vi "RT_foursetup.vi"() -> ()   [LabVIEW 2015]
uses:
  <vilib>/Platform/TimedLoop/XDataNode/timing_clust.ctl
  <vilib>/Platform/TimedLoop/XDataNode/nitl_modes.ctl
  <vilib>/Platform/TimedLoop/XDataNode/wakeup.ctl
  <vilib>/FPGAPlugInAG/myRIO-1950/niLvFpga_Open_myRIO-1950.vi
  <vilib>/rvi/interface/common/dynamic/niFpgaDynamicAddResources.vi
  <vilib>/Utility/error.llb/Error Cluster From Error Code.vi
  <vilib>/rvi/errors/niLvFpgaAdjustHostInterfaceError.vi
  <vilib>/RVI Host/nirviSupport.llb/nirviErrorClusterFromErrorCode.vi
  <vilib>/Analysis/3filter.llb/Butterworth Filter (DBL).vi
  <vilib>/rvi/interface/nirviOpenFPGA/nirviOpenFPGA.xnode
  FPGA Bitfiles/Flylaserbox_FPGATarget_FPGALASER4SETUPF_niW-GusbrOo.lvbitx
  FPGA_LASER_4SETUP_Feb19_2016.vi
  <vilib>/rvi/interface/nirviReadWriteControl/nirviReadWriteControl.xnode
  <vilib>/Platform/TimedLoop/XDataNode/XDataNode.xnode
  <vilib>/rvi/interface/nirviMethod/nirviMethod.xnode
  <vilib>/rvi/interface/Simulation/niFpgaSimulationCallBeginRW.vi
  <vilib>/Platform/TimedLoop/XDataNode/XDNodeRunTimeDep.lvlib
  <vilib>/rvi/interface/nirviMethod/StockFPGA_InlinedMethodWaitForSingleIRQ.vi
  <vilib>/FPGAPlugInAG/Dynamic/niLvFpga_WaitOnIrq_Dynamic.vi
  <vilib>/FPGAPlugInAG/Dynamic/niLvFpga_ReadFifo_Dynamic.vi
  <vilib>/rvi/errors/niLvFpgaMergeErrorWithErrorCode.vi
  <vilib>/FPGAPlugInAG/Dynamic/niLvFpga_AcknowledgeIrq_Dynamic.vi
  <vilib>/Analysis/NI_AALBase.lvlib
  NiFpgaLv.dll
panel:
  out "x-y*floor(x/y) 2":u16
  out "x-y*floor(x/y)":u16
  in  "Low Period (ticks) J8":u32
  in  "Low Period (ticks) J4":u32
  in  "Low Period (ticks) J5":u32
  in  "Low Period (ticks) J1":u32
  out "Elements Remaining 8":u32
  out "Elements Remaining 7":u32
  out "Elements Remaining 6":u32
  out "Elements Remaining 5":u32
  out "Elements Remaining 4":u32
  out "Elements Remaining 3":u32
  out "Elements Remaining 2":u32
  out "Elements Remaining":u32
  out "IRQ(s) Asserted 4":i32
  out "IRQ(s) Asserted 3":i32
  out "IRQ(s) Asserted 2":i32
  out "IRQ(s) Asserted":i32
  out "Frame Count":i16=10040
  in  "Manual control for laser":bool
  in  "Laser current control 3":u16=629
  in  "Laser current control 4":u16=629
  in  "Laser current control":u16=583
  in  "Laser current control 2":u16=629
  in  "FPGA Stop":bool
  out "Path 3":path
  out "appended path":path
  out "Path 2":path
  in  "Path":path
  out "Fly real-time location/center mass":dbl(graph)=575.5038458695241
  in  "order":i32=3
  in  "low cutoff freq: fl":dbl=40.0 format="%0.4f"
  in  "high cutoff freq: fh":dbl=400.0 format="%0.2f"
  in  "sampling freq: fs":dbl=1000.0 format="%0.2f"
  in  "threshold 3":dbl=5.0
  in  "control":u16=1
  out "Subtraction-10 frames average":dbl[](graph)=[1120.6666666666665, 1157.0, 1210.6666666666665, 1210.3333333333335, 1269.2222222222222, 1265.2222222222222, 1320.3333333333335, 1302.7777777777778, 1340.5555555555557, 1328.7777777777778, 1360.5555555555557, 1346.0, 1377.5555555555557, 1365.3333333333335, 1395.2222222222222, 1384.0, 1415.0, 1405.0, 1439.0, 1427.3333333333335, 1464.0, 1467.6666666666665, 1525.6666666666665, 1554.7777777777778, 1636.3333333333335, 1657.7777777777778, 1730.4444444444443, 1741.6666666666665, 1801.2222222222222, 1808.888888888889, 1870.3333333333335, 1880.5555555555557, 1940.3333333333335, 1944.0, 2005.0, 2002.2222222222222, 2050.0, 2039.4444444444443, 2086.4444444444443, 2082.4444444444443, 2131.777777777778, 2119.222222222222, 2166.8888888888887, 2155.4444444444443, 2197.0, 2181.8888888888887, 2225.4444444444443, 2205.8888888888887, 2243.1111111111113, 2216.4444444444443, 2259.333333333333, 2237.5555555555557, 2271.4444444444443, 2241.666666666667, 2276.777777777778, 2247.4444444444443, 2285.4444444444443, 2248.777777777778, 2285.222222222222, 2253.4444444444443, 2291.5555555555557, 2259.666666666667, 2290.666666666667, 2268.8888888888887, 2301.777777777778, 2265.4444444444443, 2306.5555555555557, 2273.8888888888887, 2306.777777777778, 2274.1111111111113, 2312.222222222222, 2278.777777777778, 2313.5555555555557, 2280.222222222222, 2316.1111111111113, 2277.666666666667, 2310.8888888888887, 2278.333333333333, 2313.777777777778, 2282.333333333333, 2305.1111111111113, 2272.0, 2304.1111111111113, 2273.333333333333, 2297.5555555555557, 2263.4444444444443, 2289.777777777778, 2257.8888888888887, 2287.0, 2246.333333333333, 2274.333333333333, 2240.4444444444443, 2264.4444444444443, 2228.333333333333, 2253.8888888888887, 2223.8888888888887, 2251.1111111111113, 2217.222222222222, 2247.0, 2214.0, 2238.4444444444443, 2201.222222222222, 2233.8888888888887, 2195.4444444444443, 2223.777777777778, 2188.777777777778, 2216.5555555555557, 2180.5555555555557, 2212.333333333333, 2176.222222222222, 2199.333333333333, 2166.666666666667, 2204.5555555555557, 2169.5555555555557, 2197.4444444444443, 2169.1111111111113, 2202.1111111111113, 2168.5555555555557, 2199.777777777778, 2173.0, 2204.5555555555557, 2160.666666666667, 2201.8888888888887, 2170.777777777778, 2197.1111111111113, 2164.0, 2186.222222222222, 2119.222222222222, 2163.5555555555557, 2179.8888888888887, 2189.4444444444443, 2190.0, 2185.1111111111113, 2187.222222222222, 2181.4444444444443, 2172.4444444444443, 2167.777777777778, 2167.0, 2149.222222222222, 2149.1111111111113, 2149.666666666667, 2153.8888888888887, 2145.0, 2149.8888888888887, 2142.777777777778, 2141.222222222222, 2137.222222222222, 2136.666666666667, 2131.0, 2131.666666666667, 2137.1111111111113, 2142.1111111111113, 2135.777777777778, 2132.666666666667, 2128.1111111111113, 2127.4444444444443, 2121.222222222222, 2122.8888888888887, 2113.4444444444443, 2114.1111111111113, 2088.333333333333, 2099.222222222222, 2110.222222222222, 2112.666666666667, 2110.0, 2112.777777777778, 2102.8888888888887, 2112.4444444444443, 2105.333333333333, 2098.5555555555557, 2103.333333333333, 2105.5555555555557, 2099.333333333333, 2087.666666666667, 2084.333333333333, 2095.4444444444443, 2091.222222222222, 2096.5555555555557, 2099.4444444444443, 2093.777777777778, 2093.333333333333, 2100.1111111111113, 2091.222222222222, 2096.0, 2094.666666666667, 2092.0, 2090.333333333333, 2084.4444444444443, 2082.222222222222, 2086.4444444444443, 2078.222222222222, 2082.0, 2083.8888888888887, 2088.777777777778, 2092.777777777778, 2090.1111111111113, 2088.222222222222, 2086.0, 2086.0, 2094.0, 2090.222222222222, 2093.333333333333, 2089.0, 2090.5555555555557, 2093.5555555555557, 2089.333333333333, 2088.222222222222, 2088.777777777778, 2092.222222222222, 2092.333333333333, 2096.4444444444443, 2096.5555555555557, 2091.5555555555557, 2094.4444444444443, 2094.0, 2095.666666666667, 2092.0, 2100.5555555555557, 2105.1111111111113, 2100.1111111111113, 2097.222222222222, 2098.8888888888887, 2096.5555555555557, 2100.1111111111113, 2107.0, 2102.222222222222, 2102.222222222222, 2097.777777777778, 2098.4444444444443, 2100.777777777778, 2099.777777777778, 2103.222222222222, 2106.4444444444443, 2109.0, 2103.1111111111113, 2110.222222222222, 2113.0, 2107.1111111111113, 2113.777777777778, 2120.0, 2121.333333333333, 2113.666666666667, 2111.0, 2108.1111111111113, 2105.8888888888887, 2105.5555555555557, 2102.8888888888887, 2104.8888888888887, 2104.666666666667, 2100.777777777778, 2105.1111111111113, 2108.5555555555557, 2104.777777777778, 2106.1111111111113, 2096.1111111111113, 2078.222222222222, 1942.888888888889, 1945.888888888889, 1952.5555555555557, 1946.111111111111, 1948.111111111111, 1945.5555555555557, 1953.0, 1959.888888888889, 1950.111111111111, 1938.0, 1953.5555555555557, 1957.2222222222222, 1962.4444444444443, 1957.111111111111, 1960.0, 1953.6666666666665, 1962.0, 1951.111111111111, 1958.0, 1961.2222222222222, 1966.5555555555557, 1967.5555555555557, 1962.3333333333335, 1965.888888888889, 1958.111111111111, 1957.3333333333335, 1957.7777777777778, 1953.2222222222222, 1958.5555555555557, 1961.111111111111, 1958.111111111111, 1963.3333333333335, 1968.0, 1965.2222222222222, 1965.888888888889, 1958.3333333333335, 1962.3333333333335, 1958.2222222222222, 1954.6666666666665, 1943.4444444444443, 1943.7777777777778, 1940.5555555555557, 1938.111111111111, 1924.7777777777778, 1930.3333333333335, 1923.4444444444443, 1914.5555555555557, 1910.111111111111, 1903.2222222222222, 1906.111111111111, 1909.5555555555557, 1894.4444444444443, 1877.6666666666665, 1863.5555555555557, 1862.0, 1839.7777777777778, 1827.2222222222222, 1850.2222222222222, 1859.111111111111, 1852.888888888889, 1870.2222222222222, 1883.888888888889, 1898.7777777777778, 1897.3333333333335, 1894.4444444444443, 1893.2222222222222, 1890.0, 1885.7777777777778, 1889.888888888889, 1893.111111111111, 1901.111111111111, 1896.7777777777778, 1900.888888888889, 1906.888888888889, 1913.888888888889, 1910.5555555555557, 1908.5555555555557, 1905.888888888889, 1906.111111111111, 1905.111111111111, 1908.2222222222222, 1897.6666666666665, 1901.2222222222222, 1904.6666666666665, 1904.0, 1902.111111111111, 1906.4444444444443, 1909.0, 1901.6666666666665, 1894.3333333333335, 1891.7777777777778, 1893.111111111111, 1895.888888888889, 1903.6666666666665, 1905.2222222222222, 1902.6666666666665, 1908.5555555555557, 1900.888888888889, 1902.5555555555557, 1897.7777777777778, 1899.6666666666665, 1896.5555555555557, 1893.4444444444443, 1886.4444444444443, 1888.3333333333335, 1889.3333333333335, 1890.7777777777778, 1891.0, 1892.4444444444443, 1890.0, 1885.0, 1880.6666666666665, 1892.111111111111, 1891.7777777777778, 1892.0, 1895.7777777777778, 1892.2222222222222, 1893.5555555555557, 1899.7777777777778, 1890.111111111111, 1890.2222222222222, 1884.2222222222222, 1884.5555555555557, 1876.2222222222222, 1877.4444444444443, 1864.6666666666665, 1860.2222222222222, 1854.7777777777778, 1946.0, 1928.6666666666665, 1965.2222222222222, 1933.888888888889, 1965.888888888889, 1939.111111111111, 1971.2222222222222, 1940.4444444444443, 1967.4444444444443, 1935.3333333333335, 1968.0, 1935.3333333333335, 1966.0, 1933.2222222222222, 1959.5555555555557, 1925.7777777777778, 1951.0, 1918.4444444444443, 1951.7777777777778, 1927.3333333333335, 1958.888888888889, 1927.3333333333335, 1944.888888888889, 1923.111111111111, 1960.6666666666665, 1925.111111111111, 1964.111111111111, 1931.7777777777778, 1958.888888888889, 1930.0, 1963.2222222222222, 1932.6666666666665, 1956.888888888889, 1924.2222222222222, 1963.6666666666665, 1934.3333333333335, 1958.4444444444443, 1932.6666666666665, 1964.0, 1932.888888888889, 1958.6666666666665, 1932.888888888889, 1964.111111111111, 1934.3333333333335, 1958.111111111111, 1930.4444444444443, 1957.2222222222222, 1928.7777777777778, 1959.3333333333335, 1921.111111111111, 1958.5555555555557, 1924.2222222222222, 1950.0, 1922.111111111111, 1948.888888888889, 1921.3333333333335, 1953.3333333333335, 1922.0, 1953.7777777777778, 1918.4444444444443, 1953.4444444444443, 1920.5555555555557, 1953.5555555555557, 1919.5555555555557, 1947.5555555555557, 1921.5555555555557, 1947.3333333333335, 1921.111111111111, 1941.4444444444443, 1913.111111111111, 1941.888888888889, 1913.7777777777778, 1938.4444444444443, 1896.888888888889, 1926.4444444444443, 1896.5555555555557, 1926.5555555555557, 1897.0, 1923.5555555555557, 1898.7777777777778, 1931.888888888889, 1899.888888888889, 1931.111111111111, 1898.4444444444443, 1934.0, 1899.4444444444443, 1933.3333333333335, 1901.7777777777778, 1937.888888888889, 1901.4444444444443, 1935.2222222222222, 1902.6666666666665, 1934.3333333333335, 1903.2222222222222, 1932.5555555555557, 1912.5555555555557, 1940.888888888889, 1904.5555555555557, 1936.0, 1904.7777777777778, 1939.888888888889, 1921.111111111111, 1938.0, 1912.3333333333335, 1936.7777777777778, 1903.888888888889, 1936.0, 1912.888888888889, 1936.7777777777778, 1904.888888888889, 1945.5555555555557, 1908.4444444444443, 1934.2222222222222, 1908.0, 1935.888888888889, 1906.0, 1934.2222222222222, 1902.4444444444443, 1931.2222222222222, 1908.0, 1938.2222222222222, 1909.0, 1936.3333333333335, 1913.3333333333335, 1945.888888888889, 1911.3333333333335, 1924.6666666666665, 1886.2222222222222, 1883.7777777777778, 1862.111111111111, 1887.6666666666665, 1874.7777777777778, 1902.6666666666665, 1875.111111111111, 1890.2222222222222, 1882.7777777777778, 1908.2222222222222, 1886.5555555555557, 1904.2222222222222, 1889.5555555555557, 1913.5555555555557, 1890.5555555555557, 1913.5555555555557, 1890.5555555555557, 1905.2222222222222, 1883.888888888889, 1912.111111111111, 1888.111111111111, 1913.888888888889, 1886.6666666666665, 1924.888888888889, 1894.0, 1915.5555555555557, 1889.4444444444443, 1910.7777777777778, 1888.5555555555557, 1909.6666666666665, 1894.888888888889, 1921.0, 1905.4444444444443, 1928.0, 1903.3333333333335, 1923.888888888889, 1900.6666666666665, 1922.888888888889, 1905.3333333333335, 1927.4444444444443, 1914.888888888889, 1929.4444444444443, 1908.888888888889, 1928.888888888889, 1901.3333333333335, 1925.0, 1906.7777777777778, 1929.6666666666665, 1908.4444444444443, 1935.888888888889, 1913.111111111111, 1934.3333333333335, 1910.3333333333335, 1927.111111111111, 1906.2222222222222, 1931.5555555555557, 1917.5555555555557, 1944.5555555555557, 1918.5555555555557, 1943.7777777777778, 1924.2222222222222, 1948.3333333333335, 1928.5555555555557, 1953.888888888889, 1937.111111111111, 1964.888888888889, 1943.888888888889, 1966.6666666666665, 1942.6666666666665, 1966.0, 1948.888888888889, 1967.6666666666665, 1942.4444444444443, 1965.3333333333335, 1943.0, 1964.3333333333335, 1949.3333333333335, 1972.7777777777778, 1947.5555555555557, 1973.0, 1950.888888888889, 1979.3333333333335, 1952.6666666666665, 1975.6666666666665, 1961.3333333333335, 1978.4444444444443, 1956.4444444444443, 1978.2222222222222, 1960.3333333333335, 1983.111111111111, 1960.0, 1985.0, 1962.7777777777778, 1984.2222222222222, 1961.7777777777778, 1986.888888888889, 1960.6666666666665, 1984.111111111111, 1958.2222222222222, 1977.6666666666665, 1961.111111111111, 1981.4444444444443, 1960.888888888889, 1980.6666666666665, 1959.6666666666665, 1980.888888888889, 1958.2222222222222, 1977.888888888889, 1961.6666666666665, 1982.3333333333335, 1964.3333333333335, 1990.0, 1972.7777777777778, 1997.3333333333335, 1970.7777777777778, 1996.888888888889, 1972.5555555555557, 1997.3333333333335, 1978.2222222222222, 1998.3333333333335, 1977.2222222222222, 2000.5555555555557, 1977.4444444444443, 2008.5555555555557, 1980.888888888889, 2003.7777777777778, 1991.3333333333335, 2001.4444444444443, 1964.3333333333335, 2019.888888888889, 1998.6666666666665, 2019.2222222222222, 2005.6666666666665, 2021.888888888889, 2013.4444444444443, 2031.111111111111, 2018.4444444444443, 2050.0, 2018.111111111111, 2044.6666666666665, 2021.6666666666665, 2044.4444444444443, 2023.6666666666665, 2050.5555555555557, 2036.2222222222222, 2054.1111111111113, 2031.3333333333335, 2059.5555555555557, 2039.0, 2056.333333333333, 2037.111111111111, 2060.4444444444443, 2049.4444444444443, 2069.8888888888887, 2044.7777777777778, 2071.4444444444443, 2053.333333333333, 2072.222222222222, 2058.4444444444443, 2080.4444444444443, 2064.777777777778, 2090.333333333333, 2067.8888888888887, 2089.333333333333, 2069.666666666667, 2093.0, 2077.666666666667, 2094.777777777778, 2076.4444444444443, 2095.0, 2075.4444444444443, 2096.8888888888887, 2079.777777777778, 2099.777777777778, 2082.5555555555557, 2102.666666666667, 2085.0, 2104.0, 2080.0, 2102.5555555555557, 2080.4444444444443, 2093.8888888888887, 2072.0, 2095.0, 2072.1111111111113, 2083.8888888888887, 2053.5555555555557, 2073.5555555555557, 2042.4444444444443, 2053.666666666667, 2022.6666666666665, 2033.0, 2003.888888888889, 2027.0, 1992.2222222222222, 2003.7777777777778, 1973.0, 1984.7777777777778, 1956.3333333333335, 1968.0, 1937.7777777777778, 1951.7777777777778, 1920.7777777777778, 1929.7777777777778, 1914.111111111111, 1917.2222222222222, 1888.2222222222222, 1889.4444444444443, 1877.7777777777778, 1889.888888888889, 1864.5555555555557, 1879.4444444444443, 1858.6666666666665, 1858.5555555555557, 1820.2222222222222, 1821.4444444444443, 1783.3333333333335, 1779.888888888889, 1742.2222222222222, 1741.2222222222222, 1708.888888888889, 1709.5555555555557, 1681.4444444444443, 1682.0, 1653.5555555555557, 1660.111111111111, 1625.4444444444443, 1620.0, 1574.2222222222222, 1554.2222222222222, 1502.6666666666665, 1484.6666666666665, 1457.3333333333335, 1458.111111111111, 1436.6666666666665, 1441.6666666666665, 1421.7777777777778, 1425.0, 1404.888888888889, 1410.5555555555557, 1381.888888888889, 1389.888888888889, 1362.5555555555557, 1372.3333333333335, 1338.7777777777778, 1346.111111111111, 1320.4444444444443, 1316.888888888889, 1272.0, 1253.0, 1206.0, 1190.7777777777778, 1151.2222222222222, 1141.888888888889, 1104.7777777777778, 1103.111111111111, 1070.3333333333335]
  in  "LED High Period (ticks) J1":u32=1520
  in  "LED High Period (ticks) J5":u32=615
  out "FIFO Timed Out? J1":bool
  out "FIFO Timed Out? J5":bool
  in  "LED High Period (ticks) J4":u32=1520
  out "FIFO Timed Out? J4":bool
  in  "LED High Period (ticks) J8":u32=1520
  out "FIFO Timed Out? J8":bool
  in  "LED stop":bool
  in  "IRQ Bit (0-31) J8":u8
  in  "Double number of pixels to take per frame J8":u16=1536
  in  "Half-clocks between frames/Trigger frequency (us) J8":u16=1600
  in  "Half-clock time/FPGA loop timer(us) J8":u32=10
  in  "Fly # 4":i32=4
  in  "Gender 4":string="F"
  in  "Date 4":string="2016Jan26"
  in  "Filename Code4":string="E1"
  in  "Fly # 3":i32=3
  in  "Gender 3":string="F"
  in  "Date 3":string="2016Jan26"
  in  "Filename Code 3":string="E1"
  in  "Fly # 2":i32=2
  in  "Fly #":i32=1
  in  "Gender 2":string="F"
  in  "Date 2":string="2016Jan26"
  in  "Filename Code 2":string="E1"
  in  "Gender":string="F"
  in  "Date":string="2016Jan26"
  in  "Filename Code":string="E1"
  out "Iteration Duration":i64=53
  in  "Wait on IRQ Timeout (ms)":i32=100
  in  "Wait on IRQ Timeout (ms) 2":i32=100
  in  "Wait on IRQ Timeout (ms) J4":i32=100
  in  "IRQ Number(s)":i32
  in  "IRQ Number(s) 2":i32
  in  "IRQ Number(s) 3":i32
  in  "FIFO Timeout setting (ms)":i32=5000
  out "Raw Data":u16[](graph)=[560, 579, 605, 604, 634, 632, 660, 652, 670, 664, 680, 673, 689, 683, 698, 692, 707, 702, 720, 714, 732, 734, 763, 777, 818, 829, 865, 871, 901, 904, 935, 940, 970, 972, 1002, 1001, 1025, 1020, 1043, 1041, 1065, 1059, 1083, 1078, 1098, 1091, 1112, 1103, 1121, 1108, 1130, 1119, 1136, 1120, 1138, 1124, 1143, 1124, 1143, 1126, 1146, 1129, 1144, 1134, 1151, 1133, 1153, 1136, 1153, 1137, 1156, 1139, 1156, 1140, 1158, 1138, 1155, 1139, 1157, 1141, 1152, 1136, 1151, 1136, 1148, 1132, 1144, 1128, 1143, 1124, 1137, 1120, 1133, 1114, 1126, 1112, 1125, 1109, 1124, 1107, 1119, 1100, 1117, 1098, 1112, 1095, 1108, 1090, 1106, 1088, 1099, 1083, 1102, 1085, 1098, 1085, 1101, 1084, 1100, 1086, 1102, 1080, 1101, 1085, 1098, 1082, 1093, 1059, 1082, 1089, 1094, 1094, 1092, 1093, 1090, 1085, 1084, 1083, 1074, 1074, 1075, 1076, 1072, 1075, 1071, 1071, 1068, 1068, 1065, 1065, 1068, 1071, 1068, 1066, 1064, 1063, 1060, 1061, 1056, 1057, 1044, 1049, 1055, 1056, 1055, 1057, 1051, 1056, 1053, 1049, 1051, 1053, 1049, 1043, 1042, 1047, 1045, 1048, 1049, 1046, 1046, 1050, 1045, 1048, 1047, 1046, 1045, 1042, 1041, 1043, 1039, 1040, 1041, 1044, 1046, 1045, 1044, 1043, 1043, 1047, 1044, 1046, 1044, 1045, 1047, 1044, 1043, 1044, 1046, 1046, 1048, 1048, 1046, 1047, 1047, 1048, 1046, 1050, 1052, 1050, 1048, 1049, 1048, 1050, 1054, 1051, 1051, 1049, 1049, 1051, 1050, 1052, 1053, 1054, 1052, 1055, 1057, 1053, 1057, 1060, 1060, 1057, 1056, 1054, 1053, 1053, 1051, 1052, 1052, 1051, 1052, 1054, 1053, 1053, 1048, 1039, 971, 973, 976, 973, 973, 972, 976, 980, 975, 968, 976, 978, 981, 978, 980, 976, 981, 975, 979, 981, 983, 984, 981, 983, 979, 979, 979, 977, 979, 981, 979, 981, 984, 982, 983, 979, 981, 979, 977, 971, 972, 970, 969, 962, 965, 961, 957, 955, 952, 953, 955, 947, 939, 931, 931, 919, 914, 925, 929, 926, 935, 942, 949, 949, 947, 947, 944, 943, 945, 946, 951, 948, 950, 953, 957, 955, 954, 953, 953, 952, 954, 949, 950, 953, 952, 951, 954, 955, 951, 947, 945, 946, 948, 952, 953, 951, 954, 950, 951, 949, 949, 948, 947, 943, 944, 945, 945, 945, 946, 945, 942, 940, 945, 946, 945, 948, 946, 947, 950, 945, 945, 942, 942, 938, 938, 932, 930, 927, 973, 964, 983, 967, 983, 969, 986, 970, 983, 968, 984, 968, 982, 967, 980, 963, 975, 959, 976, 963, 979, 964, 971, 961, 980, 962, 982, 966, 980, 965, 982, 967, 979, 962, 982, 968, 979, 966, 982, 966, 980, 966, 982, 967, 979, 965, 978, 964, 980, 960, 979, 962, 975, 961, 974, 960, 977, 961, 977, 959, 977, 960, 977, 959, 973, 961, 974, 960, 970, 956, 971, 957, 969, 948, 963, 948, 963, 949, 962, 950, 966, 950, 965, 949, 967, 949, 967, 951, 969, 951, 968, 951, 967, 952, 966, 956, 970, 952, 968, 952, 970, 961, 969, 956, 968, 952, 968, 956, 968, 952, 973, 954, 967, 954, 968, 953, 967, 951, 966, 954, 969, 955, 968, 957, 973, 955, 962, 943, 942, 930, 943, 937, 951, 937, 945, 941, 954, 943, 952, 945, 957, 945, 957, 945, 952, 942, 956, 944, 957, 943, 962, 946, 958, 945, 955, 944, 955, 947, 960, 953, 964, 951, 962, 950, 961, 953, 964, 958, 964, 955, 965, 950, 963, 954, 964, 954, 968, 957, 967, 955, 963, 953, 966, 959, 973, 959, 972, 962, 974, 964, 977, 968, 982, 973, 983, 971, 983, 974, 984, 971, 983, 972, 982, 975, 987, 973, 986, 975, 990, 976, 988, 981, 989, 978, 989, 980, 991, 980, 992, 981, 992, 981, 993, 980, 992, 979, 989, 980, 990, 981, 990, 980, 990, 979, 989, 981, 990, 982, 995, 986, 999, 986, 998, 986, 998, 989, 998, 988, 1000, 989, 1004, 990, 1002, 996, 1001, 982, 1010, 1000, 1009, 1004, 1011, 1007, 1015, 1009, 1025, 1009, 1022, 1010, 1022, 1012, 1025, 1018, 1026, 1015, 1030, 1019, 1028, 1018, 1030, 1025, 1034, 1022, 1036, 1027, 1036, 1029, 1040, 1032, 1045, 1034, 1044, 1034, 1047, 1039, 1047, 1038, 1048, 1038, 1048, 1040, 1050, 1041, 1051, 1043, 1052, 1040, 1051, 1040, 1046, 1035, 1047, 1036, 1042, 1027, 1036, 1021, 1026, 1011, 1016, 1002, 1014, 996, 1002, 986, 992, 978, 984, 969, 976, 961, 965, 957, 958, 944, 945, 939, 945, 932, 940, 930, 929, 910, 911, 892, 890, 871, 870, 855, 855, 840, 841, 827, 830, 813, 810, 786, 777, 751, 742, 729, 729, 718, 721, 711, 712, 703, 705, 691, 695, 681, 686, 669, 673, 660, 658, 636, 626, 603, 595, 575, 571, 552, 551, 535, 560, 579, 605, 606, 634, 632, 659, 649, 671, 665, 680, 672, 688, 682, 698, 691, 707, 703, 718, 712, 730, 733, 762, 778, 816, 828, 865, 871, 899, 904, 935, 938, 970, 972, 1002, 1000, 1024, 1019, 1042, 1040, 1065, 1058, 1084, 1078, 1097, 1091, 1113, 1103, 1121, 1108, 1129, 1118, 1136, 1119, 1138, 1123, 1141, 1124, 1140, 1125, 1144, 1130, 1146, 1133, 1149, 1131, 1152, 1136, 1154, 1136, 1155, 1138, 1156, 1140, 1157, 1137, 1154, 1139, 1156, 1139, 1152, 1134, 1153, 1136, 1148, 1130, 1145, 1127, 1143, 1122, 1137, 1119, 1132, 1114, 1128, 1109, 1125, 1107, 1122, 1106, 1118, 1100, 1116, 1098, 1111, 1094, 1107, 1091, 1105, 1086, 1099, 1083, 1100, 1083, 1099, 1083, 1100, 1084, 1099, 1085, 1102, 1080, 1099, 1084, 1098, 1081, 1092, 1058, 1080, 1090, 1094, 1095, 1092, 1094, 1091, 1087, 1082, 1083, 1073, 1074, 1074, 1077, 1073, 1074, 1071, 1068, 1069, 1067, 1065, 1065, 1069, 1070, 1069, 1066, 1063, 1063, 1060, 1061, 1056, 1056, 1043, 1050, 1053, 1056, 1054, 1055, 1050, 1055, 1052, 1050, 1051, 1051, 1049, 1044, 1042, 1047, 1044, 1046, 1050, 1047, 1046, 1049, 1045, 1048, 1046, 1045, 1045, 1042, 1040, 1043, 1038, 1039, 1044, 1044, 1045, 1044, 1044, 1042, 1041, 1046, 1045, 1046, 1045, 1044, 1045, 1046, 1044, 1045, 1046, 1045, 1049, 1047, 1045, 1046, 1046, 1047, 1045, 1049, 1052, 1051, 1048, 1049, 1049, 1050, 1054, 1052, 1050, 1048, 1049, 1050, 1050, 1050, 1052, 1054, 1052, 1054, 1055, 1052, 1056, 1059, 1060, 1057, 1053, 1055, 1052, 1053, 1051, 1053, 1052, 1050, 1053, 1054, 1051, 1052, 1048, 1038, 971, 972, 976, 972, 974, 973, 975, 979, 974, 970, 978, 978, 982, 977, 979, 977, 979, 974, 978, 980, 983, 983, 980, 983, 979, 978, 979, 976, 979, 979, 978, 982, 982, 984, 982, 978, 981, 978, 977, 971, 972, 970, 967, 961, 964, 962, 958, 955, 951, 952, 954, 947, 938, 932, 929, 920, 913, 924, 930, 925, 935, 941, 949, 948, 947, 946, 945, 942, 943, 946, 950, 947, 950, 953, 957, 955, 954, 953, 952, 953, 953, 948, 951, 951, 952, 951, 951, 953, 950, 947, 944, 946, 947, 949, 951, 951, 953, 951, 950, 948, 950, 946, 946, 942, 943, 945, 945, 945, 946, 943, 943, 940, 947, 945, 946, 947, 945, 945, 948, 944, 945, 943, 942, 938, 939, 931, 929, 927, 974, 962, 982, 966, 982, 969, 986, 968, 984, 966, 982, 966, 982, 965, 980, 962, 974, 959, 974, 964, 979, 963, 974, 961, 980, 962, 981, 964, 979, 965, 980, 964, 979, 960, 981, 966, 979, 967, 981, 967, 977, 964, 982, 967, 979, 965, 979, 965, 977, 960, 978, 962, 974, 960, 975, 960, 976, 961, 977, 958, 975, 959, 976, 959, 973, 960, 973, 961, 971, 956, 971, 957, 969, 950, 963, 947, 963, 947, 960, 949, 964, 950, 965, 949, 967, 949, 965, 950, 969, 950, 966, 951, 965, 950, 966, 956, 970, 953, 967, 951, 969, 958, 967, 957, 968, 951, 968, 956, 968, 952, 970, 953, 967, 954, 966, 952, 965, 950, 965, 953, 969, 953, 969, 955, 971, 955, 962, 942, 941, 932, 944, 937, 951, 938, 944, 941, 954, 943, 951, 944, 955, 945, 955, 944, 953, 941, 955, 944, 956, 942, 962, 946, 956, 943, 955, 943, 955, 947, 960, 951, 963, 952, 960, 950, 960, 951, 962, 956, 964, 954, 962, 951, 962, 952, 963, 953, 967, 956, 967, 954, 963, 952, 966, 959, 969, 959, 971, 962, 973, 964, 977, 969, 982, 970, 983, 970, 982, 973, 982, 969, 981, 970, 980, 974, 986, 974, 986, 975, 988, 977, 987, 979, 990, 978, 989, 977, 990, 978, 992, 981, 990, 979, 993, 980, 993, 979, 988, 980, 991, 978, 989, 979, 991, 978, 988, 981, 991, 982, 995, 987, 998, 984, 997, 987, 1000, 987, 999, 989, 999, 989, 1003, 991, 1001, 994, 1000, 982, 1009, 998, 1008, 1002, 1011, 1005, 1015, 1008, 1024, 1008, 1024, 1011, 1022, 1011, 1024, 1018, 1028, 1016, 1029, 1019, 1027, 1018, 1030, 1025, 1036, 1023, 1036, 1025, 1035, 1028, 1040, 1032, 1045, 1033, 1043, 1034, 1045, 1038, 1046, 1037, 1045, 1036, 1049, 1039, 1049, 1040, 1051, 1042, 1051, 1040, 1051, 1039, 1048, 1035, 1047, 1034, 1041, 1026, 1038, 1020, 1027, 1011, 1016, 1000, 1012, 995, 1001, 985, 991, 977, 982, 967, 975, 959, 963, 956, 960, 942, 944, 938, 944, 933, 938, 927, 928, 909, 910, 890, 889, 872, 871, 854, 854, 841, 839, 825, 830, 811, 810, 785, 776, 751, 742, 727, 729, 719, 720, 711, 713, 702, 704, 690, 694, 681, 687, 670, 674, 661, 658, 635, 628, 603, 596, 576, 569, 553, 551, 535, 561, 577, 605, 606, 634, 633, 660, 649, 669, 663, 681, 672, 688, 682, 697, 691, 707, 702, 720, 713, 732, 733, 761, 777, 818, 829, 865, 870, 900, 903, 934, 939, 970, 971, 1004, 999, 1023, 1020, 1044, 1040, 1065, 1058, 1084, 1076, 1098, 1091, 1112, 1103, 1121, 1107, 1129, 1117, 1133, 1122, 1138, 1122, 1141, 1123, 1142, 1127, 1145, 1128, 1146, 1132, 1150, 1133, 1152, 1136, 1152, 1137, 1156, 1139, 1156, 1139, 1157, 1139, 1154, 1138, 1156, 1140, 1151, 1135, 1153, 1135, 1149, 1130, 1144, 1129, 1143, 1120, 1136, 1119, 1130, 1114, 1127, 1109, 1125, 1107, 1122, 1107, 1118, 1100, 1115, 1097, 1111, 1091, 1108, 1091, 1105, 1087, 1098, 1084, 1102, 1083, 1099, 1082, 1099, 1085, 1099, 1085, 1102, 1079, 1099, 1085, 1097, 1080, 1092, 1057, 1080, 1090, 1094, 1095, 1092, 1092, 1090, 1087, 1083, 1082, 1074, 1076, 1074, 1077, 1072, 1075, 1070, 1069, 1069, 1067, 1066, 1066, 1067, 1070, 1068, 1065, 1063, 1063, 1059, 1059, 1057, 1056, 1042, 1049, 1054, 1056, 1053, 1055, 1051, 1057, 1052, 1049, 1052, 1052, 1050, 1043, 1041, 1048, 1046, 1048, 1050, 1047, 1046, 1050, 1045, 1046, 1046, 1044, 1046, 1043, 1040, 1041, 1039, 1042, 1042, 1044, 1044, 1045, 1043, 1042, 1042, 1047, 1046, 1045, 1045, 1045, 1046, 1044, 1044, 1044, 1045, 1045, 1048, 1049, 1045, 1045, 1046, 1045, 1046, 1049, 1051, 1049, 1048, 1050, 1047, 1049, 1052, 1049, 1050, 1048, 1049, 1049, 1048, 1051, 1052, 1053, 1050, 1053, 1054, 1053, 1056, 1058, 1059, 1055, 1054, 1053, 1052, 1051, 1051, 1051, 1051, 1048, 1051, 1053, 1051, 1052, 1047, 1039, 971, 971, 976, 973, 975, 973, 975, 980, 973, 968, 977, 979, 982, 979, 979, 977, 980, 974, 979, 979, 982, 982, 981, 982, 980, 978, 978, 976, 979, 978, 979, 981, 982, 981, 983, 978, 980, 978, 977, 971, 971, 969, 969, 962, 965, 961, 956, 954, 951, 952, 953, 945, 936, 931, 930, 919, 913, 925, 929, 926, 935, 941, 948, 947, 945, 945, 945, 942, 943, 946, 950, 948, 950, 952, 957, 954, 954, 952, 954, 952, 952, 949, 951, 951, 951, 951, 951, 953, 951, 946, 945, 947, 948, 951, 952, 951, 954, 951, 952, 949, 950, 949, 946, 942, 943, 943, 944, 945, 946, 944, 943, 940, 946, 944, 947, 948, 945, 946, 949, 944, 942, 941, 940, 936, 939, 931, 930, 926, 973, 962, 981, 967, 983, 969, 985, 970, 983, 966, 984, 966, 983, 966, 979, 961, 974, 959, 975, 963, 978, 963, 974, 961, 980, 962, 980, 966, 979, 964, 980, 965, 977, 962, 981, 966, 980, 965, 981, 966, 977, 966, 982, 968, 978, 964, 978, 964, 978, 961, 977, 962, 974, 960, 974, 961, 975, 960, 977, 960, 976, 960, 977, 960, 973, 959, 972, 960, 971, 957, 970, 955, 969, 948, 962, 947, 962, 947, 960, 947, 964, 949, 966, 950, 965, 950, 966, 951, 969, 951, 967, 950, 966, 951, 966, 955, 970, 951, 968, 950, 969, 961, 968, 955, 969, 952, 968, 957, 969, 951, 973, 954, 966, 953, 966, 951, 969, 950, 964, 954, 969, 952, 966, 955, 972, 955, 962, 942, 940, 931, 942, 937, 951, 938, 943, 940, 954, 943, 952, 943, 955, 946, 956, 945, 952, 941, 956, 943, 957, 942, 963, 947, 955, 945, 956, 944, 954, 947, 960, 952, 963, 952, 960, 948, 960, 952, 963, 956, 965, 953, 963, 950, 961, 952, 964, 955, 967, 955, 965, 954, 963, 952, 965, 957, 971, 959, 971, 961, 973, 963, 976, 968, 981, 970, 982, 971, 982, 974, 982, 971, 981, 970, 981, 973, 985, 973, 986, 975, 988, 977, 986, 979, 989, 978, 989, 979, 990, 979, 991, 981, 992, 979, 992, 979, 991, 977, 988, 979, 990, 980, 989, 977, 990, 978, 987, 980, 991, 981, 994, 985, 999, 983, 997, 986, 998, 988, 1001, 988, 1000, 988, 1003, 990, 1002, 995, 1001, 982, 1008, 997, 1009, 1001, 1010, 1006, 1015, 1009, 1024, 1007, 1022, 1010, 1021, 1010, 1025, 1017, 1027, 1015, 1028, 1019, 1028, 1018, 1030, 1023, 1034, 1020, 1036, 1025, 1035, 1029, 1039, 1033, 1044, 1033, 1045, 1034, 1045, 1036, 1046, 1037, 1046, 1035, 1049, 1039, 1049, 1040, 1051, 1041, 1051, 1039, 1050, 1039, 1048, 1036, 1047, 1034, 1041, 1026, 1036, 1020, 1026, 1010, 1016, 1000, 1013, 996, 1001, 986, 992, 977, 983, 967, 974, 959, 963, 956, 958, 943, 944, 939, 944, 933, 939, 927, 928, 909, 909, 889, 888, 870, 870, 854, 854, 841, 839, 826, 829, 812, 808, 788, 776, 751, 743, 728, 729, 718, 720, 710, 714, 701, 704, 690, 695, 681, 685, 670, 673, 661, 658, 636, 627, 603, 595, 575, 571, 553, 552, 536, 819, 846, 883, 889, 929, 931, 967, 956, 983, 977, 999, 992, 1015, 1006, 1026, 1022, 1042, 1038, 1059, 1054, 1079, 1084, 1127, 1155, 1215, 1233, 1289, 1298, 1341, 1351, 1394, 1407, 1452, 1456, 1502, 1501, 1536, 1532, 1567, 1564, 1598, 1592, 1628, 1621, 1651, 1644, 1672, 1660, 1687, 1669, 1698, 1684, 1708, 1690, 1711, 1692, 1718, 1694, 1715, 1696, 1722, 1703, 1726, 1711, 1732, 1708, 1736, 1715, 1736, 1713, 1738, 1719, 1741, 1719, 1743, 1719, 1739, 1719, 1741, 1721, 1736, 1713, 1736, 1713, 1731, 1705, 1723, 1703, 1720, 1690, 1711, 1688, 1702, 1680, 1696, 1675, 1692, 1670, 1688, 1666, 1682, 1656, 1678, 1653, 1671, 1647, 1664, 1639, 1662, 1638, 1652, 1630, 1655, 1631, 1651, 1630, 1653, 1632, 1653, 1635, 1656, 1625, 1651, 1633, 1650, 1627, 1641, 1591, 1624, 1640, 1645, 1649, 1642, 1644, 1640, 1634, 1629, 1628, 1615, 1617, 1615, 1620, 1613, 1616, 1609, 1607, 1606, 1605, 1602, 1602, 1606, 1610, 1605, 1603, 1599, 1599, 1594, 1595, 1588, 1587, 1567, 1577, 1583, 1590, 1584, 1587, 1581, 1587, 1580, 1578, 1578, 1579, 1579, 1569, 1564, 1575, 1570, 1574, 1577, 1574, 1573, 1577, 1572, 1574, 1574, 1571, 1568, 1565, 1563, 1566, 1560, 1564, 1564, 1568, 1571, 1570, 1569, 1568, 1567, 1574, 1569, 1571, 1569, 1571, 1571, 1570, 1568, 1570, 1570, 1574, 1575, 1577, 1571, 1572, 1572, 1574, 1570, 1577, 1581, 1578, 1575, 1577, 1574, 1577, 1583, 1579, 1577, 1575, 1576, 1578, 1577, 1580, 1581, 1584, 1579, 1585, 1584, 1582, 1586, 1592, 1593, 1588, 1584, 1584, 1583, 1580, 1580, 1583, 1580, 1577, 1580, 1584, 1580, 1581, 1575, 1559, 1459, 1462, 1466, 1463, 1464, 1464, 1468, 1473, 1463, 1460, 1468, 1472, 1474, 1472, 1471, 1471, 1475, 1467, 1471, 1475, 1478, 1481, 1475, 1479, 1472, 1471, 1469, 1467, 1470, 1474, 1469, 1474, 1479, 1480, 1477, 1474, 1472, 1473, 1468, 1463, 1461, 1458, 1455, 1448, 1448, 1448, 1438, 1436, 1429, 1431, 1432, 1425, 1408, 1399, 1394, 1381, 1368, 1389, 1395, 1390, 1402, 1415, 1425, 1424, 1423, 1423, 1417, 1416, 1416, 1422, 1426, 1425, 1426, 1432, 1436, 1436, 1431, 1433, 1429, 1432, 1430, 1425, 1427, 1429, 1429, 1429, 1428, 1435, 1425, 1423, 1419, 1423, 1423, 1429, 1429, 1429, 1432, 1429, 1429, 1426, 1425, 1424, 1418, 1418, 1417, 1419, 1419, 1421, 1420, 1420, 1414, 1415, 1420, 1421, 1420, 1424, 1420, 1422, 1422, 1419, 1416, 1416, 1411, 1411, 1409, 1399, 1392, 1392, 1458, 1446, 1471, 1451, 1474, 1455, 1476, 1456, 1476, 1451, 1474, 1451, 1473, 1451, 1467, 1445, 1462, 1439, 1462, 1446, 1469, 1444, 1460, 1443, 1472, 1445, 1471, 1448, 1468, 1448, 1471, 1449, 1464, 1441, 1470, 1449, 1466, 1449, 1471, 1449, 1466, 1449, 1473, 1451, 1466, 1446, 1468, 1447, 1467, 1440, 1466, 1441, 1460, 1441, 1460, 1441, 1464, 1443, 1462, 1436, 1463, 1441, 1463, 1440, 1458, 1440, 1458, 1440, 1455, 1434, 1455, 1431, 1451, 1422, 1442, 1421, 1442, 1420, 1438, 1421, 1443, 1423, 1446, 1422, 1451, 1423, 1449, 1427, 1452, 1425, 1449, 1428, 1449, 1428, 1450, 1435, 1456, 1429, 1452, 1428, 1453, 1439, 1449, 1434, 1450, 1428, 1449, 1435, 1452, 1429, 1459, 1431, 1450, 1429, 1450, 1429, 1450, 1426, 1447, 1431, 1453, 1430, 1452, 1433, 1458, 1434, 1441, 1413, 1411, 1397, 1415, 1406, 1427, 1408, 1415, 1413, 1430, 1415, 1426, 1418, 1433, 1418, 1433, 1419, 1429, 1414, 1433, 1416, 1435, 1417, 1442, 1422, 1434, 1418, 1431, 1416, 1432, 1423, 1440, 1430, 1445, 1429, 1442, 1427, 1442, 1429, 1446, 1436, 1448, 1433, 1445, 1428, 1442, 1432, 1445, 1433, 1450, 1435, 1451, 1435, 1445, 1430, 1449, 1438, 1455, 1441, 1458, 1445, 1460, 1448, 1464, 1455, 1474, 1458, 1475, 1458, 1475, 1463, 1475, 1458, 1472, 1458, 1472, 1463, 1479, 1463, 1479, 1464, 1483, 1467, 1480, 1473, 1486, 1469, 1484, 1472, 1488, 1473, 1489, 1474, 1489, 1473, 1490, 1472, 1489, 1471, 1483, 1474, 1486, 1471, 1486, 1470, 1487, 1470, 1482, 1472, 1487, 1475, 1491, 1482, 1496, 1478, 1498, 1481, 1496, 1485, 1500, 1484, 1500, 1484, 1505, 1488, 1502, 1494, 1500, 1473, 1518, 1503, 1516, 1506, 1520, 1511, 1526, 1518, 1539, 1516, 1538, 1522, 1537, 1522, 1540, 1531, 1546, 1530, 1546, 1534, 1544, 1535, 1550, 1541, 1556, 1539, 1555, 1543, 1557, 1547, 1563, 1555, 1573, 1555, 1571, 1557, 1573, 1561, 1575, 1563, 1575, 1561, 1577, 1564, 1578, 1567, 1581, 1570, 1580, 1566, 1581, 1565, 1575, 1559, 1574, 1557, 1566, 1545, 1557, 1537, 1543, 1519, 1527, 1506, 1522, 1495, 1505, 1482, 1489, 1471, 1474, 1454, 1462, 1440, 1445, 1438, 1437, 1415, 1413, 1407, 1414, 1396, 1406, 1391, 1390, 1362, 1361, 1334, 1330, 1303, 1299, 1274, 1274, 1253, 1252, 1233, 1236, 1209, 1204, 1172, 1151, 1115, 1099, 1079, 1078, 1065, 1064, 1052, 1053, 1038, 1041, 1020, 1024, 1005, 1010, 987, 991, 972, 968, 933, 918, 884, 868, 839, 830, 804, 800, 778]
  in  "FIFO Timeout setting (ms)  2":i32=5000
  out "Raw Data 2":u16[](graph)=[543, 561, 576, 584, 599, 613, 637, 667, 698, 718, 732, 740, 746, 751, 752, 756, 762, 766, 769, 770, 773, 774, 776, 780, 781, 783, 785, 791, 799, 807, 816, 829, 838, 845, 852, 857, 865, 869, 872, 878, 882, 888, 893, 899, 908, 916, 922, 931, 937, 947, 951, 959, 963, 970, 976, 983, 988, 989, 993, 996, 1001, 1004, 1006, 1008, 1010, 1010, 1013, 1016, 1018, 1017, 1018, 1019, 1018, 1018, 1018, 1019, 1018, 1020, 1019, 1022, 1020, 1022, 1022, 1022, 1022, 1024, 1020, 1022, 1022, 1019, 1020, 1019, 1017, 1013, 1014, 1014, 1012, 1008, 1006, 1007, 1004, 1003, 1001, 1003, 1000, 998, 999, 998, 994, 998, 995, 995, 992, 989, 986, 984, 978, 975, 971, 968, 968, 965, 961, 963, 963, 962, 959, 949, 955, 967, 975, 969, 966, 963, 959, 960, 960, 956, 952, 951, 950, 947, 948, 950, 949, 947, 945, 945, 945, 943, 944, 944, 941, 940, 938, 935, 933, 934, 930, 928, 927, 923, 922, 923, 921, 919, 917, 917, 915, 914, 912, 913, 911, 909, 907, 909, 906, 906, 904, 902, 901, 900, 899, 901, 900, 899, 898, 897, 897, 894, 892, 895, 893, 892, 891, 895, 892, 895, 894, 892, 894, 892, 891, 890, 886, 886, 885, 880, 880, 875, 875, 873, 874, 872, 870, 869, 869, 868, 868, 867, 863, 864, 863, 863, 863, 861, 861, 861, 859, 858, 858, 856, 856, 855, 856, 854, 855, 854, 855, 855, 857, 857, 855, 858, 858, 856, 855, 859, 860, 858, 860, 859, 858, 859, 859, 863, 841, 842, 848, 847, 853, 853, 856, 855, 862, 858, 860, 860, 859, 858, 861, 859, 858, 855, 856, 855, 856, 851, 854, 853, 852, 850, 852, 850, 849, 848, 850, 848, 851, 847, 846, 847, 848, 847, 849, 847, 848, 846, 848, 846, 849, 847, 847, 845, 847, 844, 848, 844, 846, 841, 841, 842, 845, 838, 839, 837, 839, 834, 837, 834, 836, 832, 833, 832, 833, 833, 833, 834, 835, 832, 833, 832, 834, 829, 830, 829, 832, 828, 831, 828, 829, 829, 830, 827, 829, 825, 829, 827, 831, 829, 830, 830, 832, 828, 831, 826, 826, 826, 825, 819, 822, 818, 817, 814, 816, 812, 813, 811, 812, 811, 812, 811, 809, 808, 811, 808, 811, 805, 805, 802, 803, 799, 799, 793, 804, 807, 810, 810, 810, 811, 810, 810, 811, 809, 809, 812, 809, 810, 808, 811, 812, 812, 812, 813, 814, 816, 816, 821, 821, 825, 825, 826, 827, 830, 828, 832, 828, 828, 827, 828, 822, 823, 819, 820, 817, 818, 816, 819, 814, 816, 813, 815, 812, 812, 809, 808, 804, 806, 806, 808, 806, 807, 805, 808, 810, 810, 811, 812, 811, 812, 811, 812, 812, 814, 813, 813, 809, 809, 806, 805, 801, 802, 798, 799, 798, 799, 795, 799, 797, 797, 795, 796, 796, 798, 794, 795, 794, 795, 795, 799, 799, 796, 794, 797, 797, 794, 793, 794, 793, 792, 790, 789, 789, 791, 785, 788, 788, 790, 790, 789, 785, 787, 790, 791, 792, 791, 791, 793, 787, 783, 779, 780, 806, 808, 811, 810, 806, 807, 806, 808, 807, 807, 808, 805, 806, 805, 804, 805, 806, 805, 805, 803, 802, 802, 805, 803, 807, 807, 807, 806, 806, 805, 808, 810, 809, 811, 811, 813, 814, 812, 814, 816, 816, 816, 819, 823, 826, 828, 831, 838, 842, 847, 847, 853, 855, 856, 855, 857, 857, 856, 852, 852, 848, 848, 847, 845, 845, 843, 844, 843, 842, 842, 841, 842, 842, 839, 840, 840, 838, 837, 836, 838, 840, 842, 845, 848, 850, 852, 854, 858, 858, 861, 860, 864, 864, 863, 863, 863, 864, 866, 863, 864, 863, 866, 868, 869, 870, 873, 874, 876, 878, 877, 879, 880, 881, 882, 881, 882, 883, 882, 884, 883, 882, 883, 883, 885, 887, 889, 889, 893, 924, 916, 920, 924, 928, 927, 931, 932, 937, 936, 940, 941, 948, 951, 956, 958, 962, 962, 963, 963, 963, 964, 967, 966, 972, 969, 967, 965, 966, 968, 970, 974, 980, 979, 984, 986, 992, 995, 1001, 1005, 1010, 1010, 1017, 1017, 1017, 1019, 1022, 1016, 1011, 1007, 1005, 1003, 1003, 999, 999, 999, 1000, 996, 1001, 1003, 1009, 1007, 1010, 1010, 1008, 1007, 1010, 1011, 1013, 1011, 1014, 1014, 1015, 1010, 1013, 1013, 1014, 1014, 1011, 1008, 1004, 995, 990, 981, 972, 963, 951, 941, 932, 918, 908, 894, 881, 864, 848, 828, 809, 785, 763, 741, 723, 702, 685, 666, 653, 644, 641, 637, 634, 630, 628, 625, 623, 620, 619, 615, 617, 615, 616, 615, 612, 595, 578, 558, 538, 512, 494, 479, 542, 562, 575, 584, 599, 613, 638, 666, 697, 718, 731, 741, 747, 750, 754, 757, 760, 765, 768, 769, 773, 774, 774, 778, 781, 782, 785, 790, 799, 808, 816, 829, 838, 845, 852, 858, 866, 869, 872, 878, 882, 887, 892, 900, 906, 914, 921, 930, 938, 947, 951, 959, 963, 971, 975, 984, 986, 990, 993, 997, 1001, 1004, 1005, 1008, 1011, 1009, 1013, 1016, 1019, 1015, 1017, 1019, 1018, 1019, 1017, 1018, 1019, 1020, 1018, 1022, 1020, 1022, 1021, 1024, 1021, 1024, 1019, 1021, 1023, 1021, 1019, 1018, 1016, 1014, 1014, 1015, 1010, 1007, 1008, 1006, 1003, 1003, 1002, 1002, 1000, 998, 997, 997, 993, 997, 996, 995, 990, 988, 984, 983, 979, 975, 971, 970, 967, 965, 963, 964, 963, 961, 959, 947, 955, 968, 973, 970, 967, 962, 961, 962, 959, 956, 951, 951, 949, 947, 945, 950, 949, 946, 946, 944, 944, 943, 943, 943, 943, 940, 938, 936, 932, 934, 929, 930, 928, 924, 923, 923, 920, 920, 919, 918, 916, 914, 913, 913, 911, 910, 908, 909, 906, 906, 903, 902, 901, 899, 898, 902, 899, 898, 897, 896, 897, 894, 893, 895, 894, 891, 891, 894, 892, 894, 894, 893, 894, 894, 891, 889, 886, 886, 885, 880, 881, 876, 877, 874, 873, 872, 871, 870, 870, 868, 868, 866, 865, 865, 864, 862, 863, 861, 860, 861, 859, 857, 858, 856, 856, 854, 855, 855, 855, 854, 855, 854, 858, 856, 855, 858, 859, 857, 856, 859, 860, 858, 858, 860, 858, 859, 860, 863, 843, 842, 847, 847, 853, 854, 856, 855, 860, 857, 859, 859, 859, 859, 859, 858, 857, 853, 857, 856, 854, 849, 854, 852, 853, 851, 850, 850, 849, 847, 851, 848, 850, 848, 846, 848, 849, 847, 849, 847, 847, 845, 848, 846, 850, 847, 847, 846, 847, 844, 847, 843, 846, 841, 840, 841, 845, 838, 839, 837, 839, 835, 835, 835, 837, 831, 832, 831, 834, 833, 834, 832, 834, 832, 832, 831, 834, 830, 831, 829, 831, 827, 830, 826, 830, 828, 830, 827, 830, 827, 828, 828, 830, 830, 831, 831, 832, 829, 828, 825, 827, 826, 825, 819, 823, 818, 817, 815, 814, 811, 813, 811, 813, 810, 812, 811, 808, 808, 812, 807, 810, 804, 806, 803, 803, 798, 798, 794, 805, 805, 810, 810, 810, 810, 810, 811, 809, 810, 808, 812, 809, 809, 808, 811, 810, 812, 811, 813, 814, 816, 815, 822, 821, 826, 826, 826, 829, 830, 829, 832, 828, 829, 825, 827, 822, 823, 819, 819, 818, 819, 815, 818, 814, 816, 813, 815, 811, 811, 810, 807, 805, 807, 807, 807, 806, 807, 806, 808, 809, 810, 810, 812, 810, 812, 810, 812, 814, 814, 813, 813, 810, 808, 804, 805, 801, 800, 798, 799, 797, 798, 796, 798, 797, 797, 795, 796, 795, 796, 794, 796, 794, 795, 794, 800, 799, 797, 795, 796, 795, 795, 792, 795, 793, 792, 788, 790, 791, 789, 786, 789, 788, 789, 790, 790, 785, 787, 790, 791, 792, 792, 791, 791, 786, 784, 779, 780, 806, 809, 811, 810, 807, 806, 806, 808, 808, 808, 809, 807, 806, 806, 804, 804, 807, 804, 805, 803, 802, 802, 804, 805, 807, 808, 807, 804, 807, 805, 809, 810, 810, 811, 811, 813, 814, 814, 814, 816, 816, 817, 820, 823, 825, 829, 832, 837, 840, 846, 847, 851, 855, 855, 855, 857, 857, 855, 852, 853, 848, 848, 846, 845, 845, 844, 845, 843, 842, 841, 842, 842, 842, 839, 839, 840, 838, 836, 836, 839, 841, 842, 845, 849, 851, 852, 854, 858, 857, 860, 863, 864, 865, 862, 863, 864, 863, 866, 863, 863, 863, 866, 866, 869, 871, 874, 875, 877, 879, 877, 878, 880, 882, 882, 882, 883, 881, 882, 885, 884, 882, 883, 884, 885, 886, 889, 891, 893, 925, 917, 920, 925, 928, 928, 932, 934, 939, 937, 940, 942, 948, 951, 954, 956, 963, 963, 965, 966, 964, 966, 967, 965, 970, 968, 967, 967, 967, 970, 971, 975, 981, 978, 985, 988, 991, 995, 1001, 1005, 1011, 1010, 1018, 1018, 1017, 1019, 1022, 1015, 1014, 1007, 1006, 1004, 1003, 1000, 1000, 999, 1001, 997, 1002, 1004, 1009, 1008, 1010, 1010, 1008, 1007, 1011, 1012, 1013, 1010, 1015, 1013, 1014, 1011, 1014, 1012, 1013, 1013, 1012, 1008, 1003, 996, 990, 980, 974, 962, 952, 940, 930, 918, 907, 894, 880, 864, 847, 828, 809, 783, 763, 741, 724, 702, 686, 668, 652, 645, 640, 638, 634, 631, 629, 626, 625, 619, 619, 614, 616, 615, 615, 614, 612, 596, 578, 557, 539, 511, 494, 479, 795, 822, 841, 856, 878, 902, 940, 986, 1032, 1066, 1085, 1102, 1108, 1116, 1120, 1125, 1132, 1139, 1145, 1146, 1148, 1152, 1154, 1160, 1163, 1166, 1170, 1179, 1190, 1202, 1218, 1238, 1253, 1264, 1275, 1281, 1292, 1301, 1304, 1313, 1321, 1331, 1336, 1351, 1358, 1372, 1381, 1394, 1406, 1420, 1428, 1440, 1447, 1460, 1466, 1477, 1484, 1490, 1494, 1496, 1504, 1510, 1512, 1516, 1520, 1522, 1524, 1528, 1530, 1530, 1531, 1535, 1531, 1534, 1531, 1534, 1533, 1538, 1535, 1539, 1538, 1539, 1539, 1542, 1537, 1540, 1536, 1537, 1539, 1537, 1535, 1537, 1528, 1528, 1525, 1527, 1522, 1520, 1514, 1515, 1511, 1510, 1506, 1509, 1505, 1505, 1502, 1501, 1496, 1502, 1497, 1497, 1490, 1489, 1483, 1479, 1471, 1469, 1458, 1455, 1453, 1449, 1446, 1449, 1446, 1447, 1440, 1426, 1433, 1452, 1462, 1457, 1451, 1447, 1441, 1444, 1439, 1436, 1431, 1428, 1426, 1422, 1421, 1424, 1424, 1420, 1419, 1417, 1417, 1417, 1414, 1416, 1412, 1411, 1405, 1402, 1400, 1399, 1393, 1393, 1390, 1386, 1382, 1383, 1380, 1377, 1373, 1373, 1372, 1370, 1367, 1367, 1364, 1362, 1359, 1361, 1357, 1356, 1353, 1350, 1348, 1348, 1346, 1348, 1346, 1346, 1342, 1344, 1341, 1341, 1338, 1340, 1337, 1335, 1333, 1339, 1336, 1341, 1338, 1337, 1339, 1338, 1335, 1332, 1327, 1327, 1325, 1321, 1318, 1311, 1309, 1308, 1308, 1306, 1301, 1301, 1299, 1300, 1296, 1297, 1291, 1293, 1291, 1293, 1291, 1288, 1286, 1287, 1283, 1284, 1283, 1283, 1280, 1277, 1280, 1279, 1278, 1278, 1277, 1278, 1280, 1284, 1281, 1284, 1284, 1283, 1280, 1285, 1285, 1286, 1284, 1286, 1283, 1287, 1287, 1291, 1257, 1259, 1266, 1268, 1275, 1276, 1278, 1279, 1285, 1284, 1285, 1286, 1284, 1285, 1285, 1284, 1281, 1278, 1278, 1277, 1276, 1273, 1274, 1275, 1272, 1270, 1272, 1270, 1270, 1268, 1271, 1268, 1269, 1264, 1264, 1266, 1266, 1264, 1267, 1265, 1265, 1264, 1267, 1265, 1267, 1264, 1263, 1264, 1266, 1260, 1263, 1261, 1262, 1256, 1256, 1257, 1260, 1251, 1251, 1249, 1251, 1247, 1248, 1246, 1247, 1242, 1243, 1241, 1243, 1243, 1245, 1243, 1244, 1242, 1243, 1242, 1244, 1239, 1239, 1239, 1240, 1235, 1239, 1237, 1239, 1238, 1239, 1237, 1237, 1236, 1236, 1237, 1239, 1240, 1240, 1240, 1242, 1236, 1238, 1234, 1233, 1230, 1229, 1225, 1226, 1222, 1218, 1216, 1216, 1212, 1213, 1211, 1213, 1209, 1210, 1209, 1207, 1206, 1210, 1206, 1208, 1199, 1201, 1197, 1197, 1191, 1191, 1185, 1199, 1203, 1208, 1211, 1209, 1212, 1206, 1210, 1207, 1211, 1207, 1212, 1208, 1208, 1206, 1211, 1210, 1211, 1211, 1214, 1215, 1217, 1218, 1226, 1225, 1232, 1233, 1236, 1235, 1239, 1237, 1243, 1236, 1236, 1231, 1234, 1227, 1230, 1222, 1222, 1218, 1223, 1216, 1219, 1212, 1219, 1211, 1215, 1212, 1209, 1204, 1204, 1201, 1204, 1200, 1203, 1201, 1203, 1199, 1205, 1207, 1207, 1207, 1212, 1210, 1212, 1207, 1212, 1212, 1216, 1213, 1213, 1207, 1207, 1202, 1203, 1196, 1197, 1189, 1191, 1189, 1189, 1188, 1189, 1189, 1189, 1184, 1188, 1186, 1188, 1184, 1188, 1185, 1188, 1186, 1193, 1191, 1191, 1185, 1191, 1187, 1188, 1183, 1184, 1184, 1183, 1177, 1179, 1178, 1181, 1172, 1178, 1177, 1179, 1179, 1179, 1171, 1175, 1177, 1183, 1179, 1184, 1180, 1184, 1173, 1169, 1162, 1163, 1201, 1208, 1210, 1211, 1205, 1205, 1204, 1207, 1206, 1210, 1207, 1205, 1203, 1205, 1202, 1203, 1204, 1203, 1201, 1201, 1195, 1197, 1199, 1202, 1204, 1206, 1202, 1203, 1201, 1204, 1208, 1211, 1210, 1214, 1212, 1216, 1214, 1217, 1216, 1219, 1219, 1222, 1223, 1230, 1232, 1238, 1243, 1253, 1258, 1266, 1268, 1276, 1278, 1284, 1281, 1285, 1282, 1281, 1275, 1276, 1269, 1269, 1264, 1266, 1264, 1262, 1261, 1263, 1259, 1259, 1257, 1260, 1260, 1257, 1256, 1257, 1250, 1253, 1250, 1256, 1255, 1260, 1262, 1270, 1270, 1274, 1276, 1286, 1284, 1291, 1289, 1296, 1292, 1294, 1291, 1296, 1294, 1298, 1293, 1295, 1293, 1297, 1298, 1303, 1305, 1311, 1311, 1315, 1316, 1315, 1315, 1320, 1320, 1322, 1321, 1325, 1322, 1324, 1324, 1327, 1323, 1326, 1325, 1328, 1328, 1334, 1334, 1339, 1388, 1377, 1383, 1389, 1392, 1394, 1398, 1401, 1406, 1408, 1411, 1416, 1424, 1428, 1434, 1440, 1447, 1447, 1450, 1451, 1447, 1449, 1452, 1454, 1459, 1455, 1453, 1452, 1452, 1458, 1460, 1465, 1471, 1472, 1480, 1486, 1490, 1497, 1505, 1514, 1519, 1523, 1529, 1533, 1532, 1536, 1537, 1531, 1524, 1518, 1512, 1509, 1509, 1506, 1504, 1505, 1504, 1501, 1506, 1512, 1518, 1516, 1520, 1522, 1517, 1514, 1519, 1521, 1521, 1522, 1524, 1523, 1525, 1521, 1523, 1524, 1524, 1525, 1523, 1517, 1509, 1497, 1488, 1475, 1460, 1446, 1426, 1410, 1396, 1376, 1358, 1337, 1317, 1291, 1264, 1236, 1202, 1167, 1131, 1100, 1070, 1039, 1009, 984, 959, 948, 942, 937, 931, 927, 922, 919, 917, 910, 908, 903, 903, 900, 904, 903, 898, 872, 844, 813, 783, 744, 713, 692, 542, 562, 575, 584, 600, 614, 638, 667, 698, 717, 732, 741, 747, 752, 754, 757, 762, 765, 770, 771, 773, 774, 775, 780, 782, 783, 785, 792, 800, 807, 816, 830, 839, 846, 854, 857, 866, 870, 874, 879, 882, 889, 893, 899, 908, 915, 923, 932, 938, 948, 952, 960, 964, 972, 976, 983, 988, 991, 993, 997, 1002, 1005, 1006, 1009, 1012, 1011, 1013, 1017, 1019, 1016, 1018, 1019, 1018, 1018, 1019, 1019, 1020, 1022, 1020, 1023, 1022, 1023, 1022, 1023, 1022, 1024, 1021, 1022, 1024, 1021, 1020, 1019, 1016, 1015, 1015, 1014, 1013, 1010, 1008, 1007, 1005, 1003, 1002, 1002, 1000, 999, 999, 999, 995, 997, 996, 996, 992, 990, 984, 984, 979, 978, 970, 969, 968, 965, 963, 963, 964, 963, 958, 950, 957, 967, 973, 970, 969, 964, 961, 962, 959, 957, 954, 952, 950, 947, 947, 951, 950, 946, 948, 944, 946, 945, 943, 945, 944, 940, 938, 934, 934, 936, 931, 931, 928, 926, 923, 923, 922, 919, 920, 919, 917, 915, 914, 913, 912, 910, 908, 910, 908, 907, 905, 903, 901, 902, 899, 901, 901, 900, 898, 898, 897, 896, 894, 895, 896, 891, 891, 895, 892, 895, 894, 894, 894, 894, 891, 890, 888, 886, 885, 882, 880, 878, 875, 874, 874, 874, 871, 870, 871, 870, 870, 867, 865, 866, 865, 863, 864, 861, 859, 862, 861, 859, 858, 858, 856, 856, 856, 855, 856, 856, 856, 854, 857, 857, 856, 858, 858, 857, 857, 860, 861, 857, 860, 860, 859, 860, 862, 863, 842, 845, 849, 849, 854, 854, 858, 855, 860, 859, 861, 861, 860, 860, 860, 860, 858, 856, 856, 855, 855, 850, 855, 853, 853, 851, 853, 852, 853, 849, 851, 848, 852, 847, 846, 849, 848, 847, 849, 847, 848, 846, 850, 847, 849, 848, 848, 845, 847, 845, 849, 845, 847, 841, 843, 843, 845, 838, 839, 838, 840, 835, 836, 835, 836, 833, 832, 832, 833, 833, 834, 834, 836, 834, 834, 833, 836, 829, 832, 829, 832, 828, 831, 829, 832, 829, 831, 828, 831, 827, 829, 828, 832, 831, 831, 832, 832, 828, 830, 826, 827, 826, 825, 820, 822, 819, 818, 815, 817, 812, 813, 812, 815, 811, 813, 812, 811, 809, 812, 808, 812, 805, 806, 803, 804, 799, 800, 796, 805, 807, 811, 811, 811, 811, 810, 810, 811, 811, 811, 812, 810, 810, 809, 812, 811, 812, 811, 813, 815, 817, 817, 823, 823, 827, 825, 827, 829, 832, 830, 833, 829, 830, 827, 828, 823, 824, 820, 821, 818, 820, 816, 818, 815, 816, 812, 816, 813, 811, 809, 808, 806, 807, 806, 807, 806, 808, 806, 809, 809, 810, 811, 813, 812, 811, 810, 812, 813, 815, 814, 813, 811, 809, 806, 806, 803, 802, 799, 800, 798, 799, 797, 799, 797, 797, 795, 795, 796, 796, 794, 797, 794, 796, 796, 799, 798, 798, 796, 797, 796, 796, 793, 794, 793, 793, 790, 790, 790, 791, 787, 789, 789, 791, 791, 790, 786, 788, 787, 792, 791, 792, 792, 792, 787, 784, 781, 781, 807, 808, 811, 810, 807, 806, 806, 808, 808, 808, 808, 808, 807, 806, 805, 805, 807, 805, 805, 804, 803, 803, 804, 804, 808, 808, 805, 805, 807, 806, 809, 811, 810, 812, 811, 814, 814, 814, 814, 816, 816, 817, 819, 824, 826, 829, 831, 838, 841, 847, 848, 854, 855, 855, 855, 857, 858, 856, 853, 852, 849, 849, 847, 846, 847, 845, 844, 844, 843, 843, 842, 842, 844, 839, 840, 840, 838, 837, 838, 839, 840, 843, 845, 848, 852, 852, 854, 859, 858, 860, 862, 865, 865, 864, 863, 864, 864, 865, 863, 865, 865, 865, 866, 870, 869, 873, 874, 878, 879, 877, 877, 880, 881, 881, 883, 883, 883, 882, 885, 885, 883, 884, 885, 885, 885, 888, 891, 894, 926, 917, 922, 926, 928, 928, 933, 932, 938, 937, 941, 942, 950, 950, 955, 956, 962, 961, 966, 966, 964, 964, 967, 968, 971, 967, 967, 966, 966, 970, 972, 975, 980, 979, 985, 989, 992, 994, 1001, 1006, 1011, 1012, 1018, 1018, 1018, 1019, 1021, 1015, 1013, 1008, 1005, 1003, 1002, 1002, 1002, 1000, 1002, 999, 1003, 1005, 1009, 1008, 1011, 1011, 1010, 1007, 1012, 1012, 1015, 1011, 1014, 1013, 1016, 1012, 1014, 1013, 1014, 1016, 1013, 1009, 1004, 996, 990, 981, 974, 962, 954, 941, 932, 919, 909, 896, 880, 865, 849, 829, 809, 786, 764, 743, 724, 702, 686, 667, 655, 646, 642, 638, 635, 631, 629, 626, 625, 619, 621, 615, 615, 614, 617, 617, 613, 596, 579, 558, 539, 513, 494, 480]
  in  "FIFO Timeout setting (ms)  3":i32=5000
  out "Raw Data 3":u16[](graph)=[613, 633, 659, 662, 680, 679, 702, 702, 724, 727, 745, 742, 762, 757, 770, 765, 779, 775, 790, 785, 795, 787, 804, 798, 822, 838, 870, 879, 909, 915, 940, 946, 977, 979, 1004, 1010, 1035, 1038, 1057, 1057, 1074, 1070, 1085, 1078, 1094, 1086, 1102, 1097, 1110, 1103, 1120, 1115, 1131, 1125, 1141, 1136, 1150, 1138, 1152, 1139, 1153, 1137, 1143, 1131, 1142, 1129, 1139, 1123, 1131, 1115, 1127, 1111, 1121, 1108, 1117, 1106, 1115, 1105, 1115, 1101, 1113, 1099, 1107, 1098, 1106, 1092, 1104, 1090, 1097, 1085, 1096, 1085, 1092, 1080, 1090, 1077, 1090, 1079, 1086, 1079, 1090, 1076, 1086, 1079, 1089, 1076, 1084, 1073, 1084, 1071, 1082, 1070, 1080, 1068, 1076, 1067, 1074, 1061, 1068, 1057, 1066, 1054, 1067, 1054, 1064, 1054, 1051, 1029, 1018, 1030, 1049, 1045, 1050, 1045, 1050, 1046, 1051, 1044, 1045, 1033, 1033, 1026, 1031, 1035, 1043, 1033, 1037, 1032, 1036, 1027, 1031, 1027, 1029, 1018, 1026, 1016, 1025, 1017, 1022, 1018, 1022, 1015, 1024, 1014, 1020, 1012, 1020, 1016, 1016, 1009, 1013, 1009, 1015, 1008, 1012, 1008, 1011, 1002, 1010, 999, 1004, 998, 1002, 997, 999, 991, 998, 991, 998, 990, 994, 989, 993, 985, 994, 986, 989, 984, 991, 985, 994, 985, 992, 986, 991, 985, 990, 987, 992, 984, 991, 986, 990, 983, 989, 983, 988, 979, 986, 980, 987, 980, 985, 981, 985, 979, 984, 976, 983, 977, 982, 977, 982, 978, 982, 973, 979, 972, 980, 973, 977, 969, 973, 965, 967, 964, 969, 966, 973, 966, 974, 969, 975, 966, 962, 945, 983, 995, 1001, 1003, 998, 995, 1000, 1003, 1002, 998, 999, 1001, 1001, 1001, 999, 1000, 1001, 1001, 999, 1000, 1001, 1003, 1002, 1003, 1001, 1003, 1001, 1002, 1003, 1002, 998, 998, 996, 996, 995, 995, 996, 993, 996, 997, 996, 994, 993, 993, 994, 994, 991, 992, 992, 989, 990, 987, 985, 985, 983, 984, 983, 983, 981, 980, 977, 978, 978, 977, 977, 974, 974, 971, 970, 968, 968, 967, 966, 965, 963, 959, 957, 957, 957, 957, 955, 953, 953, 952, 952, 950, 950, 950, 950, 949, 950, 949, 949, 948, 946, 949, 947, 950, 950, 951, 952, 951, 952, 953, 951, 954, 955, 952, 953, 953, 950, 953, 951, 949, 951, 949, 948, 948, 945, 947, 945, 945, 944, 943, 943, 945, 941, 934, 909, 915, 914, 913, 906, 914, 909, 912, 906, 908, 904, 907, 901, 903, 898, 906, 904, 904, 903, 905, 903, 904, 900, 903, 896, 900, 894, 899, 893, 899, 897, 901, 896, 899, 896, 900, 892, 900, 895, 900, 895, 901, 898, 901, 898, 902, 898, 905, 899, 900, 896, 899, 893, 897, 893, 896, 891, 894, 889, 891, 887, 886, 885, 885, 880, 879, 877, 878, 873, 874, 873, 877, 875, 876, 871, 879, 875, 876, 870, 877, 875, 876, 873, 876, 878, 882, 881, 886, 883, 885, 881, 883, 880, 885, 884, 890, 885, 887, 886, 888, 884, 889, 884, 891, 890, 889, 887, 890, 887, 887, 887, 889, 886, 889, 885, 890, 887, 887, 885, 888, 885, 888, 882, 888, 884, 890, 888, 886, 844, 841, 849, 844, 847, 848, 850, 847, 849, 845, 849, 845, 849, 846, 847, 845, 847, 841, 848, 842, 846, 844, 845, 843, 845, 841, 844, 838, 842, 836, 840, 837, 836, 831, 835, 831, 835, 832, 835, 830, 830, 828, 830, 827, 831, 826, 829, 825, 829, 825, 829, 823, 829, 824, 827, 824, 827, 822, 828, 824, 827, 824, 825, 824, 824, 823, 826, 821, 824, 822, 824, 819, 823, 818, 822, 820, 824, 821, 824, 823, 826, 823, 825, 819, 823, 822, 824, 820, 821, 813, 817, 815, 818, 815, 820, 816, 817, 806, 811, 808, 814, 809, 811, 814, 821, 823, 827, 825, 828, 827, 832, 829, 829, 826, 835, 836, 843, 840, 847, 845, 849, 847, 849, 841, 844, 838, 838, 842, 846, 864, 854, 869, 858, 873, 863, 878, 866, 878, 866, 880, 871, 886, 873, 892, 879, 894, 881, 899, 887, 903, 897, 914, 900, 918, 908, 925, 911, 929, 917, 937, 922, 938, 927, 945, 930, 948, 938, 952, 941, 959, 946, 966, 953, 969, 954, 972, 959, 974, 962, 982, 965, 985, 969, 988, 974, 990, 975, 994, 984, 998, 985, 1004, 988, 1003, 991, 1003, 986, 996, 978, 984, 961, 969, 952, 964, 943, 949, 935, 947, 922, 915, 894, 915, 883, 865, 824, 827, 817, 811, 781, 776, 747, 739, 713, 709, 688, 681, 658, 646, 615, 606, 589, 596, 586, 593, 582, 585, 574, 579, 561, 572, 557, 560, 548, 552, 541, 540, 524, 522, 503, 497, 478, 473, 463, 463, 450, 452, 908, 934, 969, 979, 1002, 1004, 1036, 1040, 1070, 1080, 1103, 1102, 1131, 1127, 1144, 1139, 1158, 1153, 1171, 1168, 1181, 1170, 1197, 1190, 1224, 1251, 1299, 1316, 1358, 1373, 1407, 1423, 1463, 1472, 1507, 1522, 1556, 1566, 1587, 1596, 1616, 1613, 1631, 1626, 1647, 1640, 1657, 1655, 1672, 1665, 1688, 1683, 1703, 1700, 1723, 1720, 1733, 1722, 1737, 1721, 1736, 1719, 1725, 1709, 1721, 1707, 1717, 1697, 1703, 1684, 1697, 1676, 1685, 1674, 1683, 1669, 1680, 1668, 1678, 1664, 1675, 1657, 1665, 1653, 1664, 1646, 1658, 1643, 1650, 1635, 1648, 1635, 1641, 1627, 1637, 1624, 1639, 1625, 1635, 1625, 1637, 1623, 1631, 1624, 1636, 1620, 1631, 1616, 1629, 1615, 1624, 1612, 1621, 1606, 1618, 1604, 1614, 1598, 1605, 1591, 1600, 1586, 1602, 1587, 1596, 1586, 1576, 1545, 1530, 1551, 1575, 1572, 1575, 1573, 1579, 1575, 1578, 1572, 1571, 1555, 1551, 1545, 1550, 1555, 1567, 1556, 1561, 1553, 1557, 1546, 1553, 1543, 1545, 1534, 1539, 1530, 1537, 1530, 1535, 1533, 1536, 1529, 1537, 1527, 1533, 1525, 1532, 1526, 1528, 1519, 1523, 1517, 1524, 1516, 1522, 1517, 1519, 1508, 1514, 1505, 1508, 1500, 1504, 1499, 1500, 1489, 1497, 1491, 1496, 1488, 1490, 1486, 1490, 1481, 1489, 1481, 1483, 1480, 1486, 1481, 1490, 1481, 1485, 1483, 1485, 1481, 1485, 1482, 1485, 1481, 1486, 1480, 1484, 1478, 1483, 1478, 1480, 1471, 1478, 1471, 1477, 1472, 1476, 1475, 1478, 1471, 1476, 1465, 1474, 1466, 1470, 1468, 1472, 1465, 1472, 1461, 1468, 1460, 1468, 1461, 1463, 1456, 1457, 1450, 1451, 1445, 1453, 1448, 1460, 1452, 1460, 1455, 1459, 1452, 1440, 1418, 1475, 1492, 1502, 1505, 1496, 1494, 1500, 1507, 1501, 1500, 1498, 1505, 1501, 1503, 1499, 1502, 1502, 1505, 1497, 1504, 1502, 1506, 1501, 1506, 1501, 1503, 1500, 1504, 1501, 1504, 1496, 1498, 1493, 1494, 1491, 1495, 1494, 1493, 1493, 1495, 1489, 1490, 1487, 1490, 1488, 1490, 1486, 1490, 1485, 1484, 1482, 1481, 1477, 1477, 1474, 1479, 1473, 1475, 1470, 1468, 1462, 1467, 1464, 1466, 1461, 1458, 1455, 1455, 1451, 1450, 1449, 1450, 1445, 1446, 1437, 1436, 1431, 1432, 1431, 1434, 1427, 1427, 1424, 1426, 1423, 1423, 1420, 1421, 1420, 1422, 1420, 1421, 1418, 1420, 1416, 1421, 1416, 1422, 1419, 1422, 1421, 1426, 1422, 1428, 1423, 1426, 1426, 1425, 1426, 1427, 1422, 1428, 1424, 1423, 1421, 1421, 1417, 1418, 1415, 1415, 1413, 1414, 1412, 1412, 1411, 1415, 1404, 1396, 1358, 1370, 1369, 1365, 1354, 1366, 1358, 1364, 1354, 1356, 1351, 1355, 1344, 1349, 1342, 1354, 1350, 1353, 1349, 1354, 1349, 1351, 1345, 1347, 1339, 1344, 1339, 1343, 1331, 1342, 1338, 1344, 1339, 1345, 1338, 1344, 1332, 1344, 1337, 1345, 1337, 1346, 1341, 1348, 1341, 1349, 1342, 1349, 1343, 1343, 1338, 1342, 1334, 1340, 1333, 1338, 1330, 1334, 1327, 1330, 1324, 1323, 1317, 1323, 1313, 1314, 1307, 1310, 1303, 1306, 1305, 1312, 1306, 1305, 1299, 1310, 1304, 1307, 1300, 1311, 1305, 1304, 1304, 1307, 1312, 1318, 1315, 1322, 1317, 1322, 1315, 1320, 1313, 1323, 1321, 1329, 1323, 1327, 1322, 1324, 1319, 1329, 1324, 1330, 1329, 1330, 1325, 1329, 1323, 1326, 1324, 1328, 1322, 1326, 1321, 1328, 1322, 1325, 1322, 1328, 1318, 1327, 1317, 1326, 1321, 1329, 1325, 1322, 1255, 1254, 1264, 1261, 1265, 1265, 1267, 1262, 1264, 1261, 1265, 1259, 1263, 1262, 1264, 1259, 1262, 1255, 1262, 1257, 1265, 1258, 1260, 1257, 1259, 1255, 1256, 1250, 1254, 1248, 1250, 1247, 1245, 1242, 1245, 1240, 1242, 1237, 1242, 1237, 1237, 1235, 1238, 1232, 1237, 1232, 1234, 1232, 1234, 1230, 1233, 1228, 1232, 1226, 1231, 1230, 1230, 1228, 1230, 1227, 1232, 1227, 1229, 1226, 1228, 1225, 1229, 1224, 1226, 1224, 1226, 1222, 1225, 1219, 1224, 1222, 1225, 1222, 1225, 1225, 1228, 1223, 1226, 1218, 1224, 1223, 1224, 1221, 1221, 1211, 1214, 1214, 1216, 1214, 1217, 1213, 1214, 1200, 1207, 1202, 1210, 1204, 1204, 1212, 1221, 1223, 1232, 1227, 1232, 1231, 1236, 1236, 1235, 1233, 1241, 1245, 1253, 1257, 1261, 1261, 1265, 1263, 1266, 1254, 1255, 1248, 1250, 1255, 1264, 1291, 1275, 1300, 1283, 1307, 1290, 1315, 1292, 1312, 1295, 1316, 1301, 1327, 1306, 1332, 1316, 1340, 1318, 1346, 1329, 1353, 1340, 1367, 1347, 1374, 1361, 1382, 1365, 1392, 1373, 1403, 1383, 1406, 1387, 1417, 1397, 1421, 1406, 1430, 1412, 1440, 1418, 1448, 1429, 1454, 1431, 1459, 1440, 1462, 1446, 1474, 1451, 1478, 1459, 1487, 1461, 1488, 1467, 1492, 1477, 1497, 1481, 1509, 1485, 1507, 1489, 1510, 1481, 1497, 1468, 1481, 1441, 1454, 1431, 1447, 1414, 1421, 1402, 1421, 1384, 1369, 1339, 1370, 1322, 1292, 1228, 1233, 1218, 1205, 1164, 1154, 1108, 1096, 1055, 1049, 1014, 1006, 967, 951, 902, 889, 861, 873, 858, 867, 850, 857, 839, 847, 819, 832, 811, 816, 795, 802, 787, 784, 760, 756, 730, 717, 688, 683, 665, 667, 645, 648, 613, 633, 660, 662, 682, 681, 701, 702, 725, 726, 745, 743, 763, 756, 771, 765, 780, 776, 789, 785, 795, 787, 806, 798, 822, 837, 871, 880, 911, 916, 941, 949, 976, 980, 1005, 1011, 1036, 1038, 1059, 1059, 1075, 1071, 1085, 1080, 1095, 1087, 1102, 1097, 1110, 1104, 1122, 1116, 1132, 1127, 1142, 1137, 1152, 1140, 1154, 1140, 1153, 1141, 1145, 1133, 1143, 1130, 1140, 1124, 1131, 1115, 1128, 1112, 1120, 1109, 1119, 1107, 1117, 1107, 1116, 1104, 1113, 1099, 1107, 1098, 1106, 1093, 1104, 1091, 1099, 1089, 1097, 1085, 1093, 1081, 1090, 1079, 1092, 1078, 1089, 1080, 1091, 1079, 1085, 1079, 1090, 1077, 1085, 1074, 1086, 1071, 1083, 1071, 1081, 1068, 1077, 1067, 1074, 1062, 1070, 1058, 1068, 1055, 1069, 1056, 1065, 1054, 1053, 1029, 1020, 1030, 1050, 1044, 1049, 1045, 1052, 1047, 1052, 1044, 1046, 1034, 1034, 1029, 1032, 1035, 1043, 1033, 1039, 1033, 1037, 1027, 1032, 1029, 1029, 1020, 1026, 1018, 1025, 1019, 1023, 1019, 1024, 1015, 1024, 1017, 1020, 1014, 1020, 1015, 1017, 1011, 1015, 1009, 1017, 1009, 1013, 1010, 1012, 1004, 1011, 1002, 1005, 999, 1002, 997, 1000, 992, 1000, 992, 999, 991, 994, 989, 995, 988, 995, 987, 989, 986, 992, 987, 993, 985, 993, 987, 989, 986, 991, 987, 992, 985, 992, 986, 991, 985, 989, 984, 990, 981, 987, 981, 986, 980, 985, 983, 985, 980, 987, 978, 985, 978, 983, 978, 982, 978, 981, 975, 982, 973, 981, 974, 977, 970, 974, 967, 969, 964, 970, 965, 976, 968, 974, 970, 975, 967, 962, 946, 986, 996, 1003, 1005, 1000, 995, 1001, 1005, 1001, 1000, 1001, 1003, 1005, 1001, 1002, 1002, 1003, 1002, 1002, 1000, 1003, 1003, 1003, 1004, 1003, 1003, 1002, 1002, 1003, 1003, 998, 998, 997, 997, 996, 997, 997, 995, 996, 997, 997, 996, 993, 994, 995, 992, 992, 994, 991, 991, 990, 987, 988, 984, 983, 986, 984, 982, 982, 979, 978, 978, 979, 978, 978, 975, 973, 973, 970, 968, 969, 968, 966, 965, 963, 960, 956, 957, 958, 957, 956, 954, 954, 951, 952, 951, 950, 950, 952, 951, 952, 950, 949, 950, 946, 950, 949, 950, 950, 951, 952, 953, 951, 954, 953, 953, 956, 953, 954, 953, 952, 954, 952, 949, 951, 949, 949, 948, 947, 948, 945, 944, 945, 944, 944, 945, 941, 934, 909, 918, 917, 913, 907, 914, 909, 912, 906, 907, 907, 908, 902, 904, 901, 907, 905, 906, 904, 908, 903, 906, 901, 904, 898, 901, 897, 900, 894, 900, 898, 901, 896, 899, 897, 900, 893, 899, 896, 902, 898, 901, 899, 902, 899, 903, 900, 904, 899, 900, 898, 901, 895, 899, 892, 899, 891, 895, 889, 892, 887, 887, 884, 887, 881, 881, 878, 879, 875, 876, 874, 878, 874, 876, 869, 878, 876, 878, 870, 879, 876, 876, 874, 878, 880, 883, 883, 885, 882, 886, 882, 884, 881, 886, 887, 890, 886, 887, 886, 888, 885, 890, 888, 891, 891, 891, 886, 891, 887, 888, 889, 891, 886, 890, 886, 892, 888, 889, 886, 890, 885, 888, 884, 888, 886, 891, 888, 887, 845, 842, 850, 847, 849, 847, 850, 847, 849, 847, 849, 846, 850, 846, 849, 845, 849, 841, 848, 843, 849, 845, 845, 842, 846, 842, 845, 838, 842, 837, 841, 838, 837, 832, 837, 833, 836, 831, 835, 831, 832, 828, 832, 827, 831, 827, 829, 826, 830, 825, 830, 825, 829, 825, 827, 825, 827, 823, 829, 823, 828, 825, 826, 826, 825, 823, 826, 822, 825, 824, 826, 821, 824, 820, 823, 821, 826, 822, 825, 824, 826, 824, 827, 820, 826, 822, 823, 821, 822, 815, 819, 815, 818, 815, 821, 815, 816, 807, 811, 809, 815, 810, 812, 816, 821, 823, 829, 825, 829, 826, 833, 831, 831, 827, 835, 837, 843, 843, 846, 846, 850, 848, 850, 840, 844, 837, 839, 841, 846, 866, 856, 871, 860, 875, 865, 879, 866, 877, 866, 880, 872, 888, 876, 893, 882, 895, 882, 899, 889, 905, 896, 914, 901, 919, 908, 924, 912, 930, 918, 937, 924, 939, 928, 946, 932, 951, 938, 952, 943, 961, 947, 965, 953, 969, 955, 973, 960, 975, 965, 982, 968, 986, 971, 989, 974, 992, 978, 995, 984, 999, 988, 1005, 989, 1003, 992, 1006, 988, 998, 979, 985, 962, 968, 954, 965, 945, 951, 936, 948, 923, 913, 897, 917, 885, 866, 824, 825, 818, 811, 782, 777, 748, 740, 714, 711, 688, 682, 658, 647, 615, 608, 590, 597, 587, 594, 582, 586, 574, 579, 563, 570, 558, 561, 546, 553, 542, 542, 524, 523, 503, 498, 478, 474, 462, 463, 450, 454, 613, 632, 659, 663, 681, 680, 702, 701, 724, 727, 745, 743, 763, 757, 771, 765, 781, 776, 789, 784, 795, 786, 806, 798, 822, 837, 872, 879, 909, 915, 941, 947, 974, 979, 1004, 1010, 1034, 1037, 1057, 1057, 1073, 1069, 1085, 1077, 1093, 1087, 1100, 1096, 1108, 1102, 1121, 1115, 1131, 1125, 1142, 1137, 1151, 1139, 1153, 1140, 1151, 1140, 1144, 1131, 1144, 1131, 1140, 1124, 1130, 1114, 1126, 1111, 1120, 1107, 1117, 1107, 1115, 1105, 1115, 1101, 1114, 1100, 1107, 1098, 1108, 1093, 1104, 1090, 1099, 1087, 1096, 1084, 1093, 1080, 1089, 1078, 1091, 1078, 1087, 1080, 1090, 1078, 1086, 1079, 1088, 1075, 1085, 1073, 1084, 1070, 1081, 1072, 1081, 1066, 1077, 1068, 1075, 1061, 1070, 1058, 1067, 1054, 1068, 1056, 1064, 1054, 1052, 1028, 1018, 1031, 1049, 1044, 1049, 1044, 1051, 1046, 1051, 1043, 1046, 1033, 1032, 1027, 1031, 1034, 1042, 1032, 1039, 1030, 1037, 1027, 1032, 1025, 1028, 1019, 1025, 1018, 1025, 1016, 1021, 1018, 1024, 1016, 1025, 1016, 1020, 1013, 1020, 1015, 1017, 1011, 1014, 1008, 1015, 1007, 1012, 1009, 1011, 1003, 1010, 999, 1004, 997, 1002, 995, 999, 991, 998, 992, 998, 990, 992, 988, 993, 985, 993, 985, 989, 985, 991, 986, 993, 984, 992, 986, 989, 985, 991, 988, 992, 985, 991, 985, 990, 983, 987, 985, 989, 979, 985, 979, 987, 979, 985, 981, 984, 980, 984, 978, 983, 977, 981, 978, 981, 977, 981, 973, 980, 972, 980, 974, 977, 969, 973, 966, 969, 965, 970, 965, 974, 967, 973, 968, 974, 967, 960, 947, 985, 995, 1002, 1002, 999, 996, 999, 1002, 1002, 999, 999, 1003, 1001, 1001, 999, 1001, 1001, 1000, 1000, 1001, 1001, 1002, 1001, 1004, 1002, 1002, 1002, 1002, 1003, 1002, 999, 998, 997, 996, 996, 997, 996, 993, 995, 997, 994, 994, 994, 993, 994, 994, 991, 993, 990, 990, 989, 987, 987, 986, 983, 985, 983, 982, 983, 979, 977, 978, 978, 977, 977, 973, 973, 969, 968, 967, 968, 967, 966, 965, 962, 961, 956, 955, 956, 958, 955, 953, 954, 951, 952, 951, 950, 949, 950, 949, 950, 949, 949, 948, 947, 949, 948, 950, 949, 950, 952, 954, 952, 953, 952, 952, 955, 952, 953, 953, 952, 953, 953, 950, 951, 950, 947, 948, 946, 947, 946, 945, 945, 944, 943, 944, 940, 934, 909, 915, 916, 914, 906, 913, 909, 912, 906, 906, 905, 909, 899, 903, 899, 906, 903, 904, 903, 906, 904, 906, 900, 903, 898, 899, 897, 898, 893, 898, 897, 901, 896, 899, 897, 899, 891, 900, 896, 901, 894, 900, 899, 903, 899, 903, 900, 905, 900, 900, 897, 900, 893, 897, 893, 897, 891, 894, 890, 891, 887, 887, 884, 886, 879, 880, 877, 878, 875, 874, 874, 877, 874, 875, 869, 877, 875, 875, 871, 877, 875, 875, 873, 876, 879, 882, 882, 885, 882, 885, 880, 881, 880, 886, 885, 890, 885, 888, 886, 887, 884, 889, 887, 891, 891, 891, 887, 890, 887, 888, 886, 889, 887, 889, 885, 890, 887, 887, 885, 888, 885, 887, 884, 886, 884, 892, 885, 885, 844, 842, 849, 846, 850, 848, 850, 846, 849, 846, 849, 845, 849, 845, 848, 844, 847, 842, 847, 843, 848, 843, 845, 842, 844, 841, 843, 838, 842, 837, 839, 837, 836, 832, 836, 833, 834, 832, 836, 829, 830, 828, 832, 826, 831, 826, 829, 826, 829, 824, 829, 823, 828, 825, 827, 824, 826, 822, 827, 823, 827, 825, 825, 824, 825, 823, 825, 823, 824, 823, 825, 820, 823, 819, 822, 820, 824, 820, 824, 824, 826, 823, 824, 820, 824, 821, 822, 821, 821, 813, 819, 815, 819, 816, 820, 814, 816, 807, 812, 808, 813, 810, 811, 814, 822, 822, 828, 825, 829, 826, 833, 830, 831, 825, 833, 835, 842, 842, 846, 846, 849, 847, 849, 841, 842, 836, 839, 841, 847, 864, 854, 869, 860, 874, 865, 878, 866, 877, 864, 881, 871, 888, 874, 892, 880, 895, 881, 899, 888, 903, 894, 913, 901, 917, 908, 924, 911, 930, 916, 936, 924, 939, 926, 945, 932, 950, 937, 952, 942, 960, 946, 964, 953, 969, 954, 972, 958, 974, 964, 982, 967, 984, 971, 989, 975, 992, 977, 994, 985, 1000, 986, 1004, 988, 1005, 992, 1005, 987, 997, 978, 986, 961, 969, 952, 966, 943, 948, 935, 947, 922, 914, 897, 916, 885, 866, 823, 827, 817, 809, 781, 776, 747, 739, 713, 710, 687, 681, 657, 647, 614, 606, 589, 596, 587, 592, 582, 586, 574, 580, 562, 570, 558, 561, 546, 552, 542, 540, 524, 522, 504, 496, 477, 475, 462, 463, 449, 452]
  in  "Wait on IRQ Timeout (ms) J8":i32=100
  in  "IRQ Number(s) J8":i32
  in  "FIFO Timeout setting (ms)  4":i32=5000
  out "Raw Data 4":u16[](graph)=[45, 171, 276, 331, 346, 378, 389, 405, 397, 385, 393, 412, 402, 382, 391, 397, 414, 403, 390, 396, 401, 413, 407, 396, 408, 423, 427, 404, 415, 422, 439, 430, 417, 426, 432, 444, 437, 432, 437, 438, 446, 441, 436, 443, 459, 448, 433, 442, 448, 461, 451, 439, 448, 450, 459, 451, 442, 451, 453, 460, 440, 449, 455, 468, 457, 444, 452, 456, 469, 459, 450, 457, 460, 465, 461, 453, 461, 461, 467, 448, 457, 461, 475, 465, 454, 461, 464, 473, 466, 454, 464, 465, 473, 450, 460, 465, 479, 469, 454, 462, 466, 478, 469, 458, 465, 467, 474, 467, 459, 467, 468, 474, 455, 463, 468, 482, 473, 459, 467, 470, 480, 471, 462, 470, 473, 480, 457, 463, 471, 488, 477, 461, 469, 474, 487, 476, 465, 472, 474, 482, 476, 466, 474, 476, 482, 461, 470, 474, 489, 479, 465, 473, 476, 488, 478, 471, 476, 477, 486, 464, 469, 477, 492, 483, 465, 473, 477, 492, 481, 469, 481, 483, 484, 480, 470, 479, 481, 488, 467, 475, 481, 496, 486, 471, 478, 482, 494, 484, 475, 480, 482, 493, 484, 476, 483, 499, 489, 471, 477, 483, 498, 487, 474, 481, 484, 495, 487, 475, 484, 486, 494, 472, 479, 486, 501, 491, 475, 483, 486, 500, 490, 481, 485, 488, 499, 491, 481, 488, 506, 495, 476, 484, 489, 505, 495, 481, 487, 491, 501, 494, 482, 491, 493, 501, 478, 485, 492, 507, 497, 481, 487, 492, 506, 496, 486, 490, 488, 498, 489, 478, 485, 503, 494, 474, 481, 486, 502, 493, 478, 484, 488, 500, 492, 478, 486, 490, 500, 476, 482, 489, 505, 495, 478, 483, 488, 503, 494, 486, 488, 491, 500, 493, 482, 489, 506, 498, 478, 483, 488, 505, 495, 479, 484, 488, 515, 496, 479, 487, 489, 500, 475, 479, 485, 503, 493, 475, 481, 487, 504, 494, 481, 486, 489, 499, 493, 481, 488, 491, 500, 478, 483, 489, 505, 496, 480, 486, 490, 503, 494, 479, 488, 491, 504, 478, 483, 489, 507, 498, 479, 484, 490, 506, 496, 482, 487, 491, 501, 495, 481, 489, 491, 502, 480, 485, 491, 508, 499, 482, 488, 492, 506, 497, 483, 490, 494, 506, 479, 485, 491, 508, 500, 480, 485, 490, 510, 500, 487, 492, 496, 507, 501, 487, 495, 497, 507, 483, 491, 495, 513, 503, 486, 491, 497, 510, 502, 490, 495, 497, 511, 485, 489, 495, 514, 504, 486, 491, 496, 513, 504, 489, 494, 498, 503, 499, 488, 496, 499, 509, 486, 491, 498, 514, 506, 487, 494, 497, 511, 511, 496, 497, 500, 513, 503, 491, 498, 516, 507, 487, 492, 497, 516, 505, 490, 495, 499, 511, 503, 488, 497, 498, 510, 485, 491, 496, 515, 505, 488, 492, 498, 513, 503, 491, 496, 498, 513, 502, 490, 497, 516, 507, 487, 492, 497, 515, 506, 489, 495, 498, 512, 502, 489, 497, 500, 511, 487, 492, 499, 516, 508, 489, 494, 498, 515, 505, 493, 497, 500, 513, 504, 492, 499, 516, 507, 486, 491, 496, 515, 505, 489, 494, 498, 512, 503, 488, 497, 501, 513, 486, 492, 498, 516, 507, 489, 493, 498, 515, 506, 495, 497, 499, 510, 503, 492, 498, 516, 508, 488, 493, 499, 517, 508, 491, 496, 500, 514, 505, 489, 498, 501, 514, 489, 494, 501, 519, 507, 488, 494, 499, 517, 506, 492, 497, 501, 525, 510, 495, 502, 503, 514, 491, 497, 502, 519, 510, 494, 498, 503, 517, 508, 493, 502, 504, 518, 491, 497, 503, 521, 512, 493, 497, 503, 519, 510, 494, 500, 503, 514, 507, 495, 502, 504, 515, 492, 496, 502, 520, 512, 494, 499, 503, 518, 508, 495, 502, 505, 517, 492, 497, 504, 521, 514, 493, 499, 503, 522, 512, 497, 502, 506, 516, 512, 497, 505, 507, 518, 495, 501, 506, 524, 515, 498, 504, 508, 522, 513, 502, 507, 509, 523, 498, 500, 507, 526, 517, 499, 503, 509, 525, 516, 501, 507, 510, 517, 513, 501, 510, 513, 522, 499, 505, 511, 527, 519, 501, 508, 512, 526, 516, 506, 510, 513, 525, 515, 503, 512, 528, 519, 499, 505, 509, 526, 515, 499, 504, 508, 520, 510, 509, 509, 508, 518, 492, 498, 502, 520, 511, 493, 497, 501, 515, 507, 494, 498, 499, 514, 502, 488, 494, 511, 502, 480, 482, 487, 504, 495, 476, 478, 481, 495, 486, 467, 471, 471, 486, 460, 460, 465, 482, 477, 457, 458, 460, 478, 471, 456, 455, 458, 474, 465, 446, 450, 465, 460, 435, 434, 435, 453, 448, 48, 161, 219, 278, 320, 375, 386, 380, 392, 397, 417, 395, 397, 402, 421, 418, 400, 401, 405, 423, 419, 404, 423, 420, 437, 412, 415, 422, 443, 438, 420, 424, 431, 450, 444, 428, 434, 437, 451, 445, 431, 439, 442, 449, 430, 436, 444, 461, 453, 436, 441, 445, 461, 452, 440, 444, 448, 460, 452, 439, 446, 463, 456, 436, 441, 445, 465, 455, 439, 443, 448, 460, 453, 438, 446, 448, 461, 436, 442, 447, 465, 456, 440, 444, 448, 463, 455, 442, 447, 447, 461, 452, 440, 446, 465, 456, 436, 440, 446, 463, 454, 437, 443, 446, 460, 451, 436, 444, 446, 458, 434, 438, 444, 461, 454, 436, 439, 443, 461, 451, 440, 442, 446, 459, 451, 437, 444, 461, 454, 434, 439, 444, 463, 454, 437, 441, 444, 459, 451, 434, 442, 445, 459, 434, 437, 444, 460, 452, 434, 437, 442, 459, 451, 438, 450, 450, 457, 450, 436, 443, 459, 454, 432, 437, 442, 461, 452, 435, 439, 443, 457, 450, 433, 441, 443, 457, 432, 435, 442, 459, 452, 432, 436, 440, 458, 449, 434, 437, 441, 454, 447, 433, 439, 443, 454, 432, 435, 440, 457, 451, 433, 437, 442, 457, 449, 431, 440, 442, 457, 431, 435, 441, 459, 453, 433, 437, 442, 459, 450, 435, 439, 443, 455, 449, 434, 441, 444, 456, 432, 437, 442, 459, 453, 435, 439, 443, 459, 450, 435, 441, 444, 459, 432, 436, 443, 461, 453, 434, 437, 442, 460, 452, 435, 440, 443, 455, 445, 428, 435, 438, 450, 426, 429, 434, 453, 445, 429, 432, 436, 453, 445, 431, 434, 437, 453, 428, 430, 436, 454, 447, 427, 430, 435, 453, 446, 429, 432, 437, 449, 443, 427, 434, 437, 444, 423, 428, 434, 452, 445, 428, 432, 435, 451, 442, 428, 431, 434, 450, 440, 425, 429, 463, 447, 424, 426, 430, 450, 442, 426, 429, 433, 448, 441, 424, 431, 433, 448, 423, 427, 433, 450, 444, 426, 429, 433, 450, 442, 428, 430, 433, 448, 439, 425, 431, 450, 443, 422, 425, 430, 449, 441, 425, 427, 431, 447, 439, 423, 429, 432, 445, 421, 424, 430, 448, 442, 423, 425, 429, 447, 440, 426, 429, 432, 448, 439, 425, 430, 449, 443, 421, 425, 429, 447, 440, 425, 428, 434, 449, 441, 424, 432, 435, 450, 424, 427, 432, 451, 443, 424, 427, 432, 449, 442, 427, 431, 433, 445, 440, 425, 432, 450, 444, 423, 427, 432, 451, 443, 425, 429, 432, 448, 440, 423, 430, 434, 448, 423, 426, 432, 451, 443, 423, 426, 431, 449, 440, 426, 429, 432, 444, 439, 424, 431, 432, 446, 421, 425, 437, 455, 443, 426, 428, 433, 447, 440, 422, 430, 432, 447, 420, 425, 431, 448, 442, 422, 425, 430, 448, 440, 423, 427, 430, 444, 437, 422, 428, 431, 443, 420, 423, 429, 446, 440, 422, 425, 430, 446, 438, 421, 427, 431, 446, 420, 423, 429, 447, 441, 420, 423, 429, 447, 438, 423, 426, 430, 442, 437, 421, 429, 431, 444, 419, 422, 426, 444, 438, 420, 424, 428, 444, 436, 424, 427, 430, 446, 420, 423, 428, 446, 439, 419, 422, 428, 445, 438, 421, 425, 428, 442, 435, 419, 426, 430, 436, 416, 421, 427, 445, 439, 420, 424, 429, 445, 437, 424, 426, 429, 445, 435, 421, 428, 446, 439, 418, 423, 427, 446, 438, 422, 425, 429, 443, 436, 420, 428, 430, 443, 419, 423, 429, 447, 439, 421, 425, 431, 452, 440, 426, 429, 431, 446, 436, 423, 430, 449, 441, 421, 425, 430, 448, 440, 422, 427, 430, 445, 437, 421, 429, 431, 444, 419, 422, 429, 446, 439, 420, 423, 428, 445, 437, 425, 426, 431, 445, 437, 422, 429, 447, 441, 419, 424, 428, 447, 439, 422, 426, 430, 445, 437, 420, 429, 432, 446, 421, 425, 431, 450, 441, 423, 426, 432, 448, 440, 427, 431, 433, 445, 438, 425, 432, 450, 443, 423, 427, 432, 450, 442, 425, 430, 433, 447, 440, 425, 432, 435, 448, 423, 427, 434, 451, 443, 424, 428, 433, 450, 441, 427, 431, 435, 446, 440, 426, 433, 435, 446, 423, 427, 433, 449, 442, 424, 428, 431, 445, 438, 421, 429, 430, 445, 418, 422, 427, 446, 438, 418, 420, 425, 443, 434, 419, 421, 425, 436, 430, 414, 420, 422, 434, 426, 420, 421, 436, 429, 409, 411, 414, 430, 422, 404, 408, 410, 425, 397, 399, 403, 422, 416, 395, 396, 400, 419, 413, 394, 395, 399, 412, 406, 387, 393, 394, 409, 382, 381, 384, 403, 397, 377, 376, 37, 148, 228, 303, 335, 347, 364, 376, 396, 391, 373, 380, 385, 400, 374, 378, 385, 403, 396, 378, 381, 387, 406, 399, 389, 393, 399, 411, 407, 395, 404, 423, 417, 397, 404, 410, 429, 419, 404, 410, 415, 428, 420, 420, 421, 421, 432, 406, 414, 420, 438, 427, 411, 416, 422, 436, 427, 413, 420, 423, 433, 426, 416, 423, 425, 432, 411, 418, 423, 438, 429, 414, 421, 423, 437, 427, 413, 423, 426, 436, 410, 417, 425, 441, 432, 412, 419, 423, 440, 429, 417, 421, 424, 433, 428, 415, 423, 425, 435, 411, 418, 423, 440, 430, 415, 420, 424, 437, 428, 413, 422, 424, 437, 410, 417, 423, 441, 431, 413, 418, 423, 440, 427, 415, 421, 424, 435, 427, 414, 423, 426, 436, 413, 419, 424, 441, 432, 415, 420, 424, 438, 429, 418, 423, 425, 437, 412, 417, 423, 441, 433, 412, 418, 423, 440, 431, 416, 420, 424, 434, 427, 414, 422, 425, 433, 411, 417, 424, 440, 431, 414, 420, 424, 437, 429, 418, 422, 425, 438, 428, 416, 423, 442, 432, 412, 418, 424, 441, 432, 416, 420, 424, 436, 429, 414, 422, 425, 435, 422, 425, 426, 442, 434, 415, 421, 424, 440, 431, 419, 423, 426, 440, 430, 418, 425, 444, 434, 414, 420, 426, 442, 433, 418, 422, 426, 438, 431, 416, 424, 426, 437, 413, 419, 425, 442, 434, 417, 420, 426, 441, 432, 421, 424, 426, 440, 430, 418, 425, 444, 435, 414, 420, 425, 443, 433, 417, 417, 421, 434, 427, 411, 419, 422, 435, 409, 413, 420, 438, 430, 411, 415, 420, 437, 428, 415, 419, 422, 432, 427, 414, 420, 438, 431, 410, 415, 420, 438, 429, 413, 417, 421, 434, 427, 411, 419, 421, 434, 409, 413, 419, 437, 429, 409, 413, 418, 434, 426, 411, 414, 417, 429, 423, 408, 415, 418, 429, 406, 410, 416, 433, 427, 408, 428, 423, 434, 425, 409, 417, 420, 433, 408, 412, 419, 436, 428, 409, 413, 417, 435, 426, 411, 415, 418, 430, 424, 409, 416, 419, 430, 406, 411, 416, 434, 426, 409, 413, 417, 432, 424, 407, 415, 418, 432, 406, 410, 416, 434, 426, 406, 410, 415, 433, 421, 408, 413, 417, 429, 423, 407, 415, 418, 429, 405, 409, 418, 435, 428, 410, 416, 420, 435, 426, 414, 417, 421, 434, 409, 413, 419, 437, 429, 408, 413, 418, 436, 426, 411, 415, 420, 431, 425, 409, 418, 419, 430, 407, 412, 418, 436, 427, 410, 414, 419, 434, 425, 413, 418, 420, 435, 424, 412, 418, 437, 427, 408, 412, 417, 435, 426, 409, 414, 418, 432, 423, 410, 417, 419, 430, 407, 411, 418, 434, 427, 409, 405, 425, 436, 424, 413, 415, 419, 432, 423, 410, 417, 435, 427, 407, 411, 416, 435, 425, 410, 413, 418, 430, 423, 407, 416, 418, 431, 404, 410, 416, 434, 426, 407, 411, 416, 432, 423, 411, 414, 417, 432, 421, 408, 415, 435, 426, 405, 409, 416, 433, 425, 407, 413, 416, 430, 422, 406, 413, 416, 429, 403, 408, 415, 432, 424, 406, 410, 414, 431, 422, 410, 413, 416, 427, 421, 407, 415, 432, 426, 404, 410, 414, 433, 423, 407, 411, 415, 429, 421, 406, 414, 416, 430, 403, 408, 415, 433, 424, 406, 409, 415, 431, 422, 408, 412, 415, 427, 421, 408, 415, 417, 427, 404, 409, 414, 432, 424, 406, 412, 415, 430, 422, 407, 415, 418, 430, 404, 410, 416, 434, 425, 406, 411, 416, 433, 423, 409, 412, 417, 427, 422, 407, 415, 413, 434, 407, 412, 417, 433, 426, 409, 414, 418, 431, 424, 408, 416, 418, 432, 405, 410, 416, 435, 425, 406, 411, 417, 433, 422, 408, 413, 417, 429, 422, 408, 415, 418, 429, 405, 410, 416, 433, 425, 408, 413, 416, 432, 423, 412, 415, 419, 432, 406, 411, 419, 436, 428, 407, 413, 417, 435, 425, 411, 416, 420, 431, 424, 410, 418, 421, 430, 407, 414, 420, 437, 428, 411, 416, 421, 435, 426, 415, 419, 422, 435, 424, 414, 420, 439, 429, 409, 414, 421, 437, 428, 412, 418, 421, 433, 425, 411, 419, 422, 432, 408, 412, 419, 435, 426, 408, 414, 418, 432, 422, 411, 414, 417, 430, 420, 407, 413, 432, 423, 402, 406, 411, 430, 420, 404, 408, 412, 424, 415, 399, 407, 407, 420, 393, 397, 418, 426, 413, 395, 396, 400, 415, 407, 391, 392, 394, 410, 401, 385, 391, 409, 403, 381, 384, 388, 407, 399, 380, 382, 386, 401, 393, 373, 377, 379, 394, 367, 367, 372, 389, 37, 168, 247, 281, 316, 349, 381, 381, 363, 367, 373, 392, 384, 367, 372, 375, 389, 383, 368, 376, 379, 392, 369, 375, 383, 402, 397, 380, 387, 393, 409, 401, 391, 397, 401, 413, 390, 394, 403, 421, 412, 393, 401, 406, 423, 413, 400, 406, 410, 418, 413, 400, 409, 421, 422, 398, 407, 412, 428, 418, 403, 409, 413, 426, 417, 407, 413, 415, 427, 417, 408, 414, 432, 420, 403, 409, 414, 429, 420, 405, 412, 415, 426, 418, 406, 414, 416, 424, 402, 408, 415, 430, 421, 404, 411, 413, 428, 418, 408, 413, 415, 426, 418, 407, 414, 431, 421, 401, 409, 413, 430, 420, 404, 411, 415, 426, 418, 405, 414, 416, 426, 401, 409, 415, 432, 421, 404, 408, 414, 429, 420, 410, 414, 416, 428, 420, 408, 415, 433, 423, 402, 410, 415, 432, 421, 406, 412, 415, 428, 419, 405, 414, 416, 428, 402, 409, 415, 431, 422, 404, 409, 414, 430, 420, 410, 413, 416, 425, 419, 407, 415, 432, 424, 403, 409, 414, 432, 421, 406, 411, 415, 428, 419, 405, 414, 429, 430, 403, 409, 416, 433, 423, 405, 411, 415, 432, 421, 408, 413, 417, 426, 420, 408, 416, 417, 427, 404, 409, 415, 431, 422, 407, 413, 416, 429, 421, 405, 415, 417, 429, 403, 409, 415, 434, 424, 405, 411, 415, 431, 422, 408, 414, 417, 427, 421, 408, 416, 418, 428, 405, 412, 416, 433, 424, 408, 414, 418, 431, 423, 409, 416, 419, 431, 404, 411, 417, 430, 421, 401, 406, 411, 428, 419, 404, 409, 413, 423, 417, 403, 411, 414, 423, 400, 405, 411, 428, 420, 403, 409, 412, 427, 417, 406, 410, 413, 427, 401, 405, 412, 430, 421, 401, 406, 411, 428, 418, 403, 408, 411, 421, 415, 401, 409, 411, 422, 397, 403, 409, 425, 416, 398, 403, 407, 422, 413, 402, 406, 409, 424, 414, 403, 408, 427, 417, 397, 402, 408, 425, 416, 399, 419, 414, 424, 414, 400, 408, 411, 422, 397, 402, 409, 426, 417, 400, 405, 409, 424, 415, 403, 407, 410, 423, 414, 402, 408, 427, 417, 397, 402, 406, 425, 415, 399, 404, 408, 421, 413, 397, 406, 408, 420, 395, 400, 407, 425, 415, 397, 401, 406, 421, 413, 400, 403, 406, 422, 413, 402, 409, 428, 419, 399, 404, 410, 427, 417, 401, 406, 410, 423, 414, 400, 408, 411, 423, 397, 403, 409, 427, 417, 399, 404, 408, 425, 415, 405, 407, 410, 420, 415, 401, 409, 425, 420, 397, 403, 408, 427, 416, 400, 405, 409, 422, 415, 398, 407, 409, 422, 396, 402, 408, 426, 416, 398, 402, 409, 424, 415, 400, 405, 408, 419, 413, 400, 408, 410, 418, 396, 400, 406, 423, 415, 397, 403, 406, 435, 416, 399, 406, 410, 421, 395, 401, 408, 425, 417, 396, 403, 406, 424, 413, 400, 404, 408, 418, 413, 399, 406, 409, 419, 395, 401, 406, 423, 414, 398, 402, 407, 420, 412, 397, 405, 407, 420, 394, 400, 405, 424, 415, 395, 400, 405, 421, 412, 396, 401, 405, 416, 409, 395, 403, 406, 417, 394, 399, 405, 422, 413, 396, 402, 405, 420, 411, 400, 404, 407, 419, 395, 398, 405, 423, 414, 394, 400, 406, 422, 412, 397, 402, 406, 416, 410, 396, 404, 407, 417, 393, 399, 405, 422, 413, 397, 401, 406, 419, 412, 399, 404, 406, 420, 410, 399, 405, 424, 414, 395, 400, 406, 423, 413, 397, 403, 407, 419, 411, 397, 404, 408, 418, 395, 399, 407, 423, 414, 397, 403, 407, 422, 411, 416, 410, 410, 421, 412, 400, 407, 425, 416, 396, 401, 407, 424, 414, 399, 403, 408, 419, 412, 397, 406, 408, 419, 394, 401, 407, 424, 414, 397, 402, 407, 421, 413, 400, 405, 408, 420, 411, 400, 407, 425, 415, 396, 401, 407, 424, 414, 398, 405, 407, 421, 412, 399, 407, 410, 420, 396, 402, 409, 425, 416, 399, 404, 409, 424, 415, 404, 408, 411, 420, 414, 403, 410, 427, 420, 398, 405, 410, 428, 417, 402, 408, 411, 423, 415, 400, 410, 412, 424, 397, 405, 410, 428, 418, 399, 405, 410, 425, 416, 401, 407, 410, 419, 413, 400, 407, 410, 417, 395, 400, 406, 422, 413, 396, 402, 405, 418, 410, 394, 402, 404, 416, 389, 396, 402, 419, 411, 390, 394, 398, 414, 403, 389, 392, 395, 405, 406, 391, 395, 394, 405, 379, 382, 386, 403, 394, 376, 379, 383, 399, 391, 374, 379, 382, 397, 370, 373, 378, 397, 389, 368, 370, 374, 390, 380, 362, 364, 365, 379, 372]
  in  "IRQ Bit (0-31) J4":u8
  in  "Double number of pixels to take per frame J4":u16=1536
  in  "Half-clocks between frames/Trigger frequency (us) J4":u16=1600
  in  "Half-clock time/FPGA loop timer(us) J4":u32=10
  in  "IRQ Bit (0-31) J5":u8
  in  "IRQ Bit (0-31) J1":u8
  in  "Double number of pixels to take per frame J5":u16=1536
  in  "Half-clocks between frames/Trigger frequency (us) J5":u16=1600
  in  "Half-clock time/FPGA loop timer(us) J5":u32=10
  in  "Stop FPGA data acquisition":bool
  in  "Double number of pixels to take per frame J1":u16=1536
  in  "Half-clocks between frames/Trigger frequency (us) J1":u16=1600
  in  "Half-clock time/FPGA loop timer(us) J1":u32=10
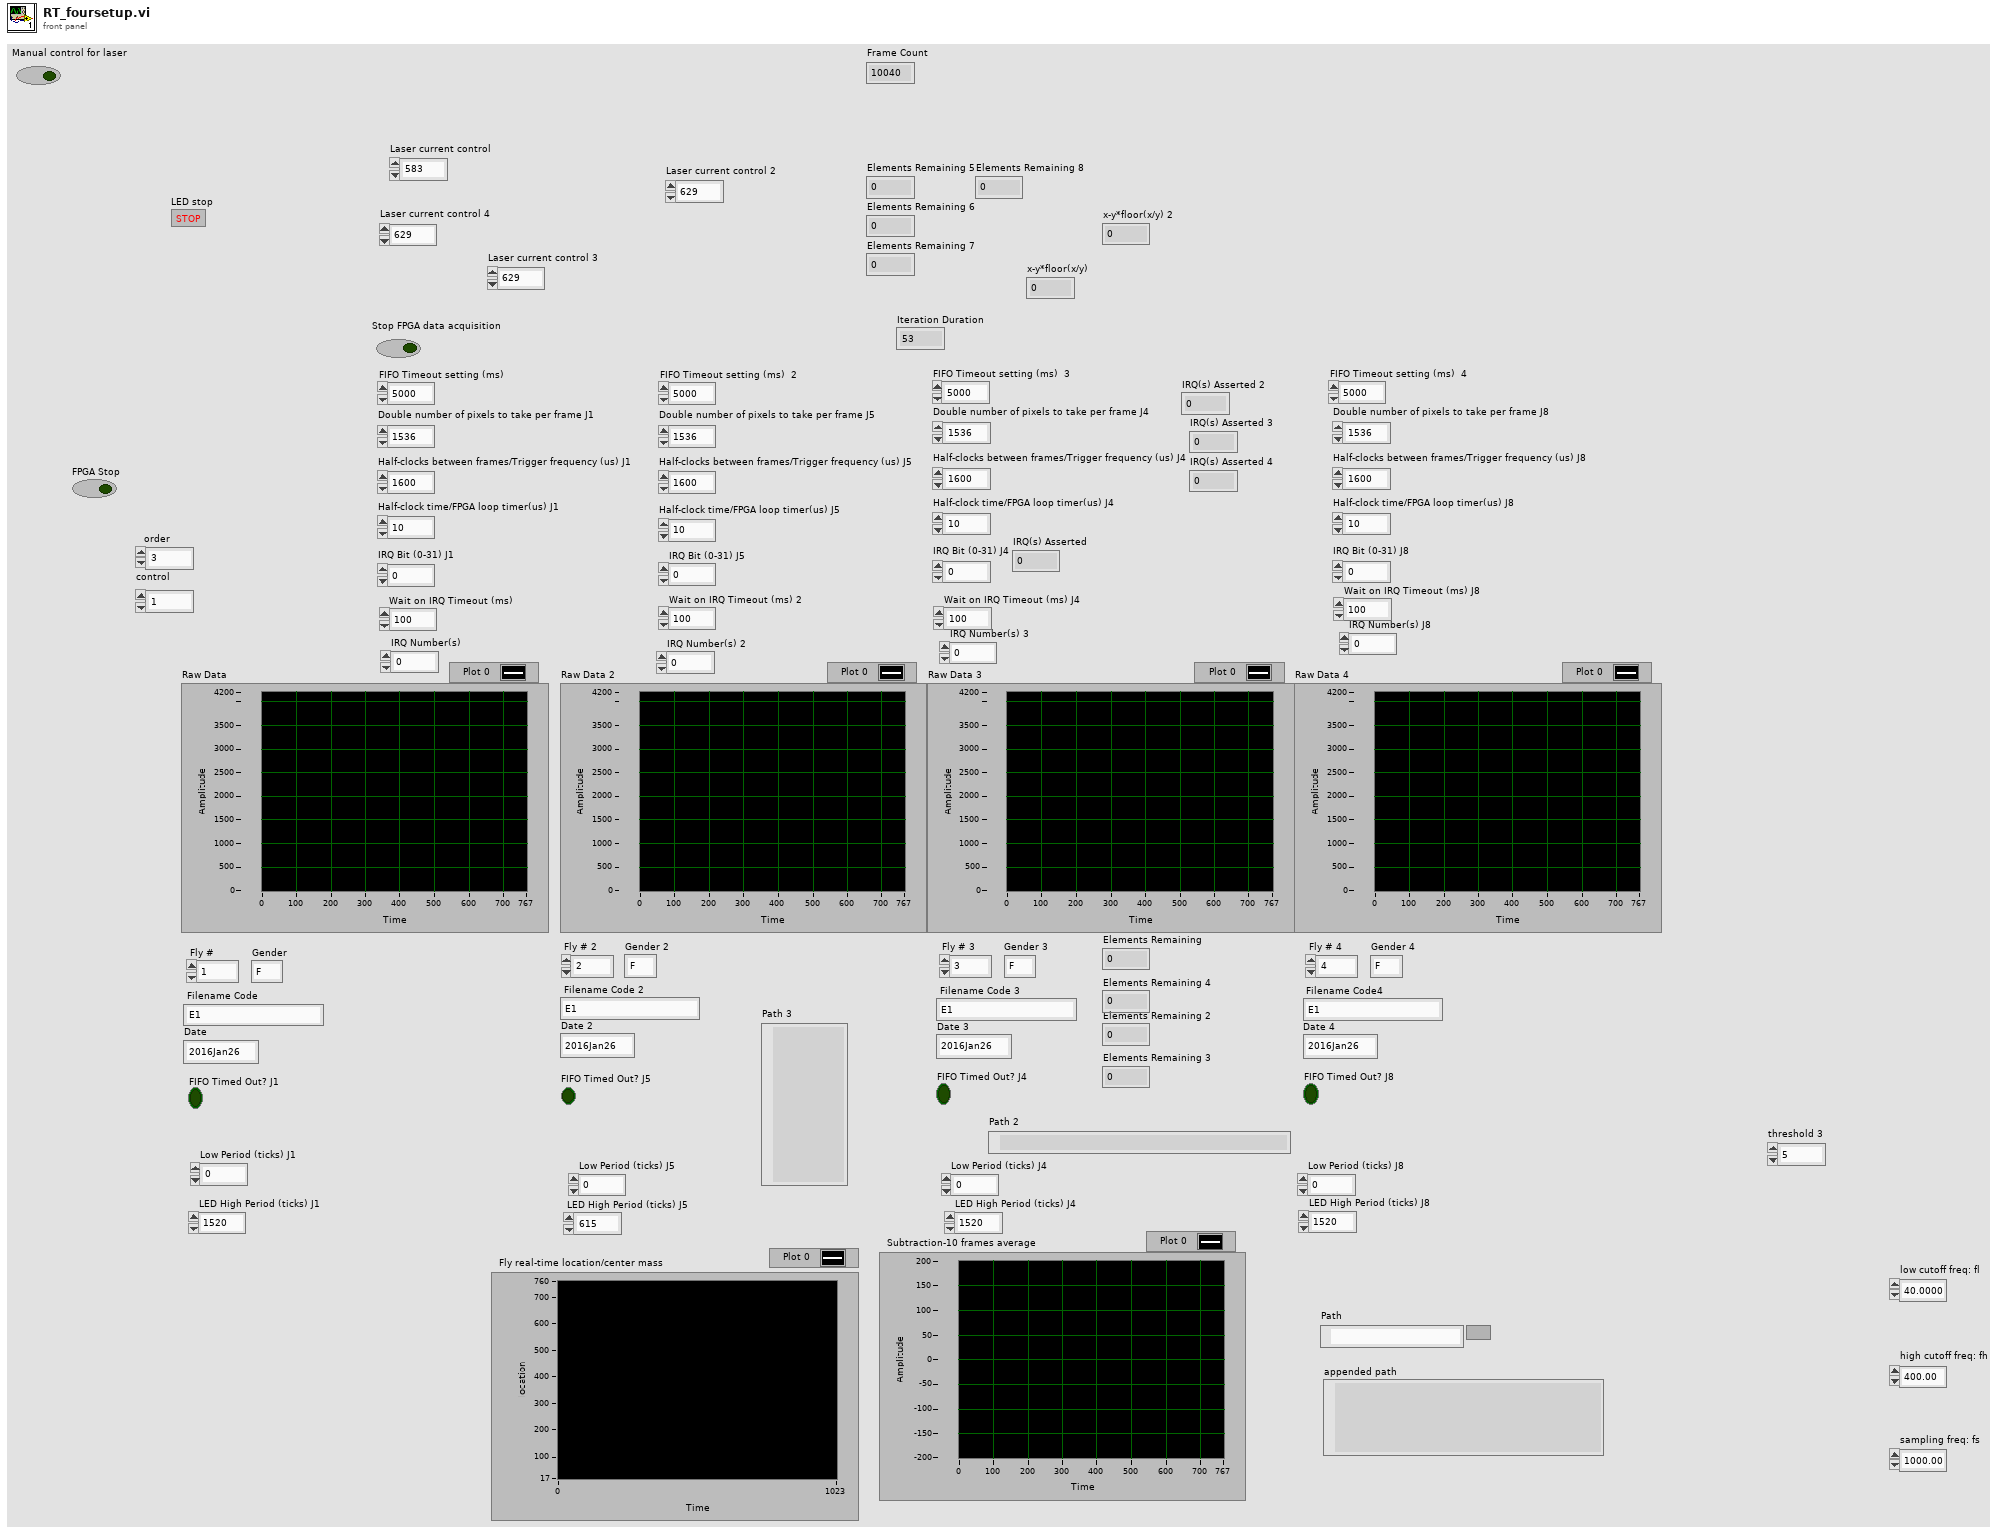
[diagram p1: front panel]
types:
  T1 = enum16{"open", "open or create", "create or replace", "create", "open (read-only)"}
  T2 = typedef "XDNodeRunTimeDep.lvlib/timing_clust.ctl" = cluster{"Expected End [f-1]":u64, "Actual End [f-1]":u64, "Finished Late? [f-1]":bool, "Expected End [i-1]":u64, "Actual End [i-1]":u64, "Finished Late? [i-1]":bool, "Expected Start [i]":u64, "Actual Start [i]":u64, "Expected Start [f]":u64, "Actual Start [f]":u64, "Source Name":string, "Structure Name":string, "Period":i64, "Deadline":i64, "Offset":i64, "Start":i64, "Priority":i32, "Timeout":i32, "Mode":T3, "Wakeup Reason":T4, "Error":errorcluster, "Source Type":string, "Secondary Source Type":string, "Global End Time":u64, "Global Start Time":u64, "Frame Duration":u64, "Iteration Duration":u64, "Assigned CPU":i32, "I/O Scan Engine Mode":u32}
  T3 = typedef "XDNodeRunTimeDep.lvlib/nitl_modes.ctl" = enum32{"No Change", "Process missed periods, maintain original phase", "Discard missed periods, maintain original phase", "Process missed periods, ignore original phase", "Discard missed periods, ignore original phase"}
  T4 = typedef "XDNodeRunTimeDep.lvlib/wakeup.ctl" = enum32{"Normal", "Aborted", "Asynchronous wakeup", "Timing source error", "Timed loop error", "Timeout"}
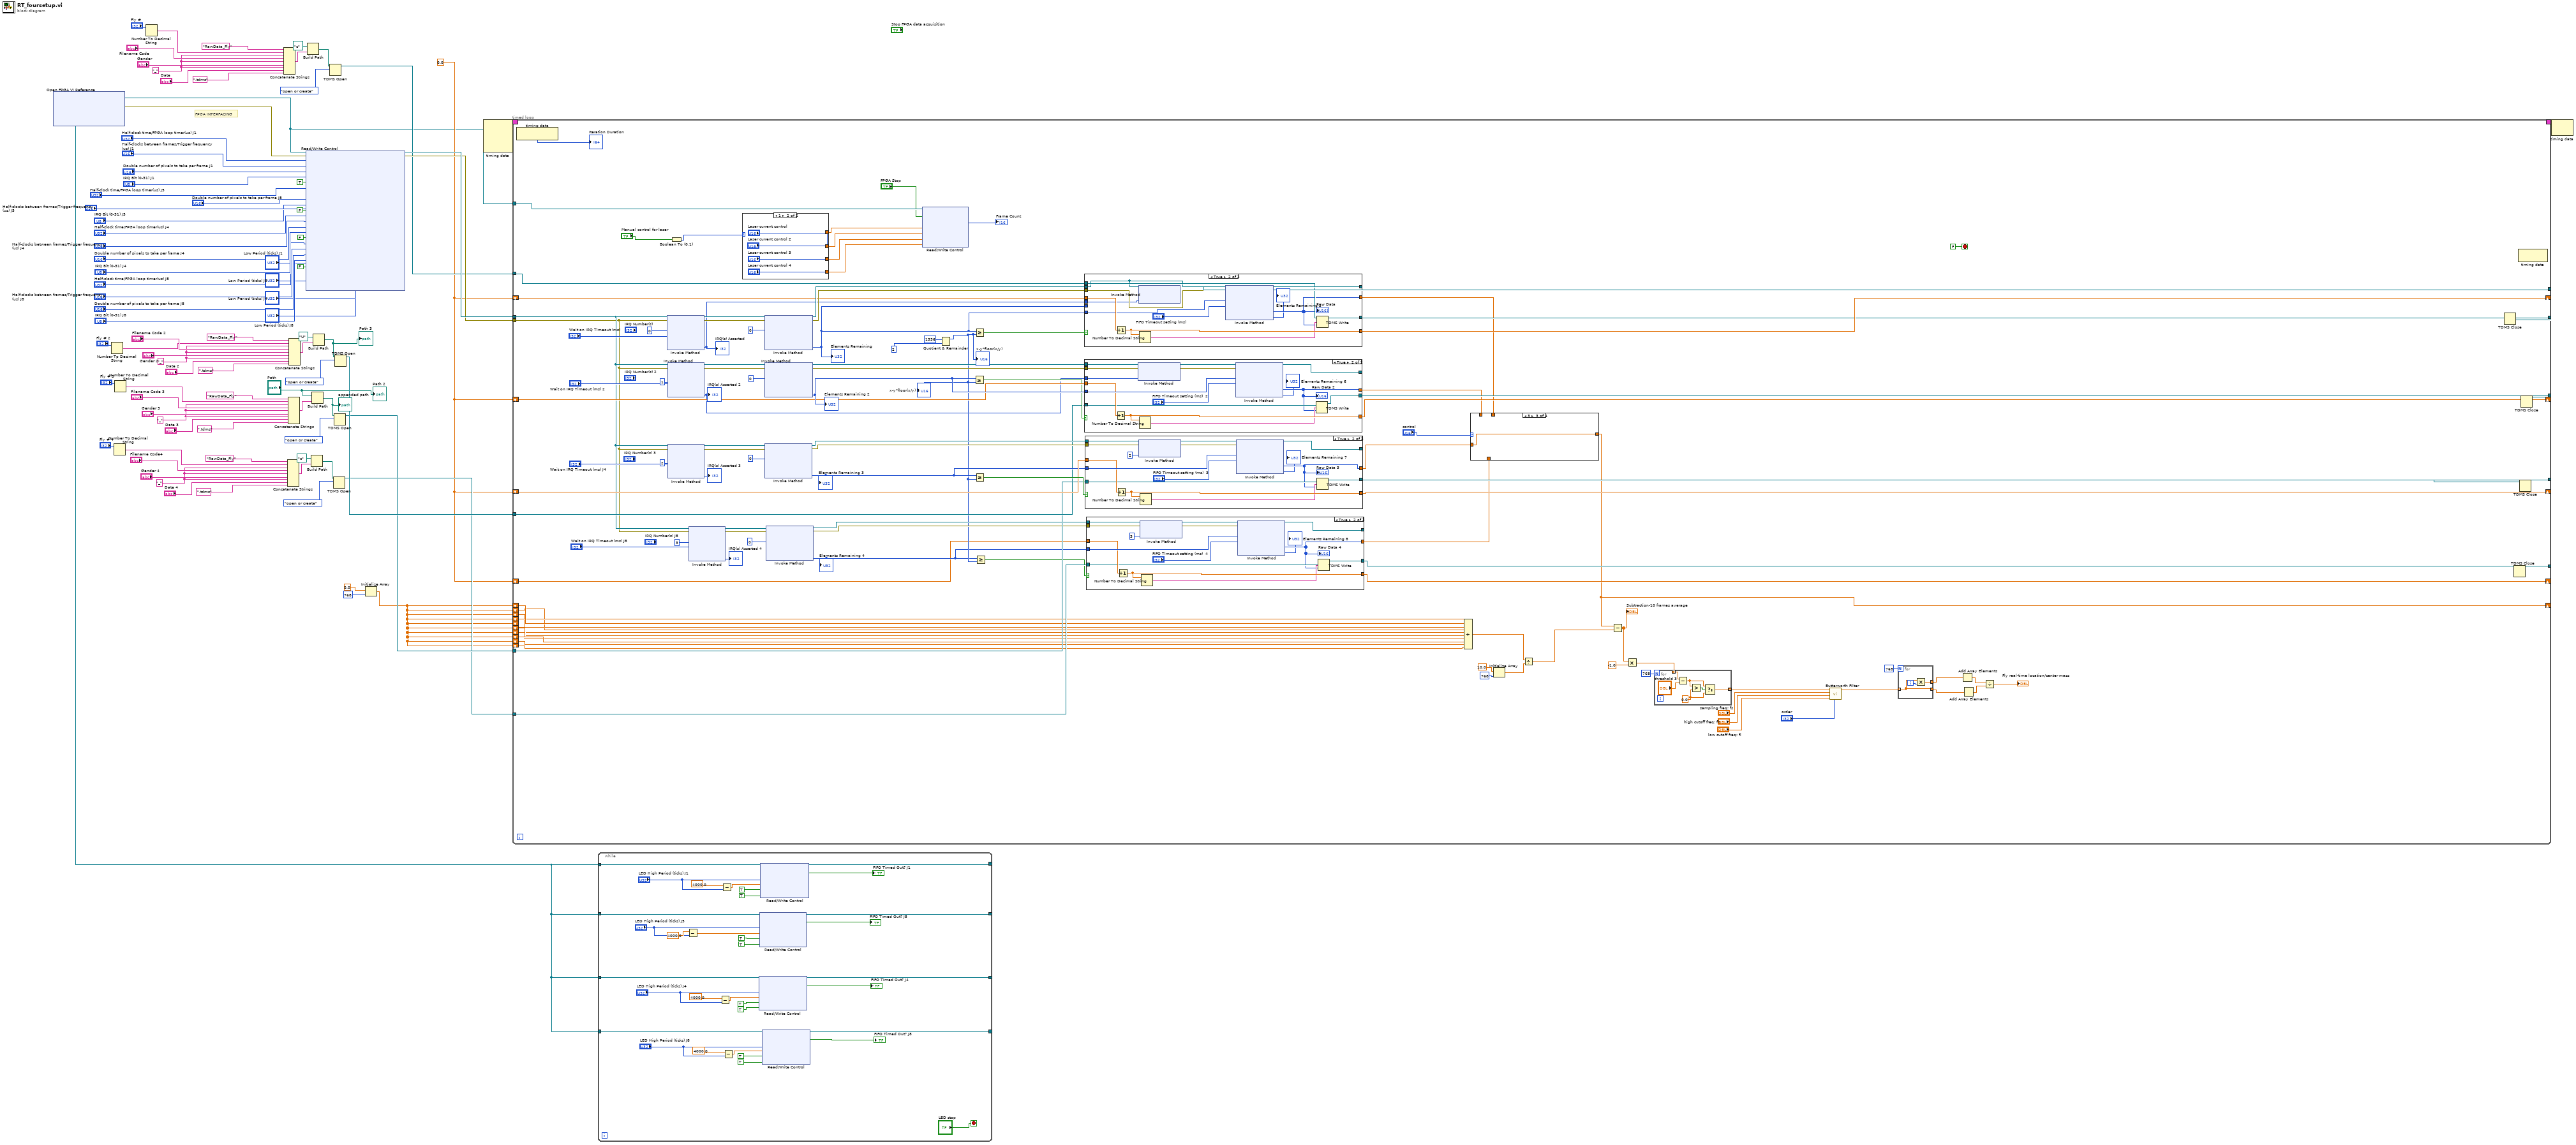
[diagram p0: block diagram]
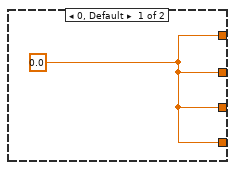
[diagram p2: hidden frame]
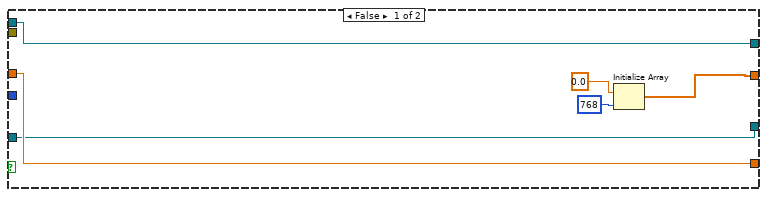
[diagram p6: hidden frame]
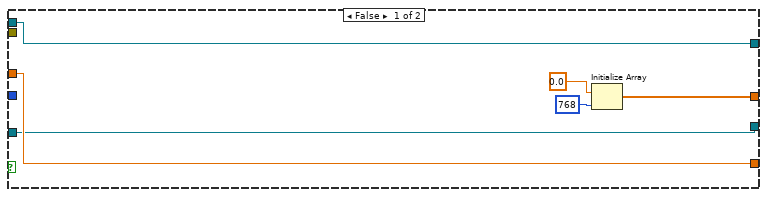
[diagram p7: hidden frame]
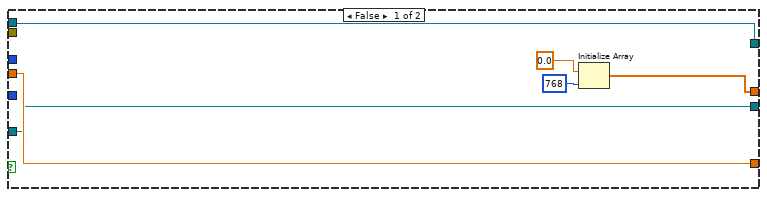
[diagram p8: hidden frame]
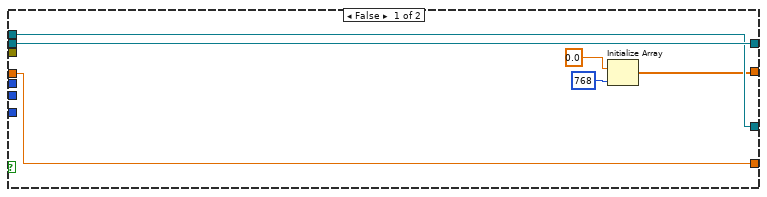
[diagram p9: hidden frame]
diagram:
  w22 = "_" ("string")
  w37 = "_" ("string")
  w51 = "_" ("string")
  w62 = "_" ("string")
  w12 = 0.0
  # "FPGA INTERFACING"
  n1 = xnode "Open FPGA VI Reference"() -> ("FPGA VI Reference Out"=w5:refnum<k20>, "error out"=w88:errorcluster)  [unwired: 2 in]
  n2 = Number To Decimal String(number="Fly # 2") -> (decimal integer string=w45:string)  [unwired: 1 in]
  n3 = Number To Decimal String(number="Fly # 4") -> (decimal integer string=w19:string)  [unwired: 1 in]
  n4 = Number To Decimal String(number="Fly # 3") -> (decimal integer string=w34:string)  [unwired: 1 in]
  n5 = Number To Decimal String(number="Fly #") -> (decimal integer string=w47:string)  [unwired: 1 in]
  n6 = Concatenate Strings("RawData_Fly" ("string"), w47, w62, "Filename Code", w62, "Gender", w62, "Date", ".tdms" ("string")) -> (w66:string)
  n7 = Concatenate Strings("RawData_Fly" ("string"), w19, w22, "Filename Code4", w22, "Gender 4", w22, "Date 4", ".tdms" ("string")) -> (w26:string)
  n8 = Concatenate Strings("RawData_Fly" ("string"), w34, w37, "Filename Code 3", w37, "Gender 3", w37, "Date 3", ".tdms" ("string")) -> (w41:string)
  n9 = Concatenate Strings("RawData_Fly" ("string"), w45, w51, "Filename Code 2", w51, "Gender 2", w51, "Date 2", ".tdms" ("string")) -> (w55:string)
  n10 = xnode "Read/Write Control"("FPGA VI Reference In"=w5, "error in"=w88, "Half-clock time J1"="Half-clock time/FPGA loop timer(us) J1", "Half-clocks between frames J1"="Half-clocks between frames/Trigger frequency (us) J1", "double number of samples to take per frame J1"="Double number of pixels to take per frame J1", "IRQ Bit (0-31) J1"="IRQ Bit (0-31) J1", "Wait Until IRQ Cleared? J1"=TRUE ("Wait Until IRQ Cleared?"), "Half-clock time J5"="Half-clock time/FPGA loop timer(us) J5", "Half-clocks between frames J5"="Half-clocks between frames/Trigger frequency (us) J5", "double number of samples to take per frame J5"="Double number of pixels to take per frame J5", "IRQ Bit (0-31) J5"="IRQ Bit (0-31) J5", "Wait Until IRQ Cleared? J5"=FALSE ("Wait Until IRQ Cleared?"), "Half-clock time J4"="Half-clock time/FPGA loop timer(us) J4", "Half-clocks between frames J4"="Half-clocks between frames/Trigger frequency (us) J4", "double number of samples to take per frame J4"="Double number of pixels to take per frame J4", "IRQ Bit (0-31) J4"="IRQ Bit (0-31) J4", "Wait Until IRQ Cleared? J4"=FALSE, "Half-clock time J8"="Half-clock time/FPGA loop timer(us) J8", "Half-clocks between frames J8"="Half-clocks between frames/Trigger frequency (us) J8", "double number of samples to take per frame J8"="Double number of pixels to take per frame J8", "IRQ Bit (0-31) J8"="IRQ Bit (0-31) J8", "Wait Until IRQ Cleared? J8"=FALSE ("Wait Until IRQ Cleared? J4"), "Low Period (ticks) J1"="Low Period (ticks) J1", "Low Period (ticks) J5"="Low Period (ticks) J5", "Low Period (ticks) J4"="Low Period (ticks) J4", "Low Period (ticks) J8"="Low Period (ticks) J8") -> ("FPGA VI Reference Out"=w72:refnum<k20>, "error out"=w71:errorcluster)
  n11 = Build Path(base path=path "c:/", name or relative path=w66) -> (appended path=w69:path)
  n12 = Build Path(base path=path "c:/", name or relative path=w26) -> (appended path=w29:path)
  n13 = Build Path(base path="Path", name or relative path=w41) -> (appended path=w43:path)
  "appended path" <- w43
  n14 = Build Path(base path=path "U:/", name or relative path=w55) -> (appended path=w6:path)
  "Path 3" <- w6
  n15 = TDMS Open(10:T1."open or create" ("operation (0:open)"), 11:w69) -> (3:w60:refnum<k34>)  [unwired: 5 in, 1 out]
  n16 = TDMS Open(10:T1."open or create" ("operation (0:open)"), 11:w29) -> (3:w18:refnum<k34>)  [unwired: 5 in, 1 out]
  n17 = TDMS Open(10:T1."open or create" ("operation (0:open)"), 11:w43) -> (3:w32:refnum<k34>)  [unwired: 5 in, 1 out]
  n18 = TDMS Open(10:T1."open or create" ("operation (0:open)"), 11:w6) -> (3:w49:refnum<k34>)  [unwired: 5 in, 1 out]
  n19 = Initialize Array(0.0 ("element"), 768 ("dimension size")) -> (w8:dbl[])
  n20 = node-c288() -> (w90:T2)  [unwired: 4 in]
  n21 = timed-loop {
    timing: w90 -> [_]
    timing-out: [_] -> w89
    tunnel: w72 -> [w156]
    tunnel: w71 -> [w155]
    tunnel: [w185] -> _
    shift-right: [w180] -> _
    shift-left: w12 -> [w181]
    shift-right: [w175] -> _
    shift-left: w12 -> [w176]
    shift-right: [w168] -> _
    shift-left: w12 -> [w170]
    tunnel: w60 -> [w166]
    tunnel: [w165] -> w59
    tunnel: w49 -> [w164]
    tunnel: [w163] -> w33
    tunnel: w32 -> [w162]
    tunnel: [w161] -> w31
    tunnel: w18 -> [w150]
    shift-right: [w148] -> _
    shift-left: w12 -> [w149]
    tunnel: [w147] -> w11
    shift-right: [w128] -> _
    shift-left: w8 -> [w145]
    shift-left: w8 -> [w137]
    shift-left: w8 -> [w138]
    shift-left: w8 -> [w139]
    shift-left: w8 -> [w140]
    shift-left: w8 -> [w141]
    shift-left: w8 -> [w142]
    shift-left: w8 -> [w143]
    shift-left: w8 -> [w144]
    shift-left: w8 -> [w111]
    tunnel: w5 -> [w108]
    stop <- FALSE stop-if-true
    n22 = node-c288() -> (→"Iteration Duration":i64)  [unwired: 1 in]
    n23 = xnode "Invoke Method"("FPGA VI Reference In"=w156, "error in"=w155, "IRQ Number(s)"=0, "Timeout (ms)"="Wait on IRQ Timeout (ms)") -> ("FPGA VI Reference Out"=w199:refnum<k20>, "error out"=w196:errorcluster, "IRQ(s) Asserted"=w93:i32)  [unwired: 1 out]
    "IRQ(s) Asserted" <- w93
    n24 = xnode "Invoke Method"("FPGA VI Reference In"=w156, "error in"=w155, "IRQ Number(s)"=1, "Timeout (ms)"="Wait on IRQ Timeout (ms) 2") -> ("FPGA VI Reference Out"=w198:refnum<k20>, "error out"=w195:errorcluster, "IRQ(s) Asserted"=w92:i32)  [unwired: 1 out]
    "IRQ(s) Asserted 2" <- w92
    n25 = xnode "Invoke Method"("FPGA VI Reference In"=w156, "error in"=w155, "IRQ Number(s)"=2, "Timeout (ms)"="Wait on IRQ Timeout (ms) J4") -> ("FPGA VI Reference Out"=w197:refnum<k20>, "error out"=w194:errorcluster, "IRQ(s) Asserted"=→"IRQ(s) Asserted 3":i32)  [unwired: 1 out]
    n26 = Boolean To (0,1)(Boolean="Manual control for laser") -> (0, 1=w101:i16)
    n27 = xnode "Invoke Method"("FPGA VI Reference In"=w156, "error in"=w155, "IRQ Number(s)"=3, "Timeout (ms)"="Wait on IRQ Timeout (ms) J8") -> ("FPGA VI Reference Out"=w160:refnum<k20>, "error out"=w159:errorcluster, "IRQ(s) Asserted"=→"IRQ(s) Asserted 4":i32)  [unwired: 1 out]
    n28 = case shown="1" w101 {
      tunnel: [w201 "Laser current control"] -> w104
      tunnel: [w201 "Laser current control 2"] -> w103
      tunnel: [w201 "Laser current control 3"] -> w106
      tunnel: [w201 "Laser current control 4"] -> w105
      frame 0, Default {
        w201 = 0.0 ("y")
      }
      frame 1 {
      }
    }
    n29 = xnode "Invoke Method"("FPGA VI Reference In"=w197, "error in"=w194, "Number of Elements"=u32 0) -> ("FPGA VI Reference Out"=w174:refnum<k20>, "error out"=w173:errorcluster, "Elements Remaining"=w169:u32)  [unwired: 1 in, 1 out]
    "Elements Remaining 3" <- w169
    n30 = xnode "Invoke Method"("FPGA VI Reference In"=w199, "error in"=w196, "Number of Elements"=u32 0) -> ("FPGA VI Reference Out"=w187:refnum<k20>, "error out"=w186:errorcluster, "Elements Remaining"=w91:u32)  [unwired: 1 in, 1 out]
    "Elements Remaining" <- w91
    n31 = xnode "Invoke Method"("FPGA VI Reference In"=w198, "error in"=w195, "Number of Elements"=u32 0) -> ("FPGA VI Reference Out"=w178:refnum<k20>, "error out"=w177:errorcluster, "Elements Remaining"=w179:u32)  [unwired: 1 in, 1 out]
    "Elements Remaining 2" <- w179
    n32 = xnode "Invoke Method"("FPGA VI Reference In"=w160, "error in"=w159, "Number of Elements"=u32 0) -> ("FPGA VI Reference Out"=w154:refnum<k20>, "error out"=w153:errorcluster, "Elements Remaining"=w151:u32)  [unwired: 1 in, 1 out]
    "Elements Remaining 4" <- w151
    n33 = xnode "Read/Write Control"("FPGA VI Reference In"=w108, "FPGA Stop J1"="FPGA Stop", "ConnectorB/AO0 J1"=w103, "ConnectorA/AO0 J5"=w104, "ConnectorB/AO1 J4"=w106, "ConnectorA/AO1 J8"=w105) -> ("Frame Count J1"=→"Frame Count":i16)  [unwired: 1 in, 2 out]
    n34 = Quotient & Remainder(x=u16 1536, y=u16 2) -> (x-y*floor(x/y)=w152:u16)  [unwired: 1 out]
    "x-y*floor(x/y)" <- w152
    "x-y*floor(x/y) 2" <- w152
    n35 = Greater Or Equal?(x=w179, y=w152) -> (x >= y?=w172:bool)
    n36 = Greater Or Equal?(x=w91, y=w152) -> (x >= y?=w182:bool)
    n37 = Greater Or Equal?(x=w169, y=w152) -> (x >= y?=w171:bool)
    n38 = Greater Or Equal?(x=w151, y=w152) -> (x >= y?=w146:bool)
    n39 = case shown="True" w172 {
      tunnel: w178 -> [w265 w281]
      tunnel: [w265 w278] -> _
      tunnel: w179 -> [_ w277]
      tunnel: w176 -> [w266 w275]
      tunnel: [w266 w274] -> w175
      tunnel: w177 -> [_ w272]
      tunnel: w164 -> [w264 w271]
      tunnel: [w264 w270] -> w163
      tunnel: [w261 w269] -> w132
      tunnel: w92 -> [_ w267]
      frame False {
        n40 = Initialize Array(0.0 ("element"), 768 ("dimension size")) -> (w261:dbl[])
      }
      frame True {
        n41 = Increment(x=w275) -> (x+1=w274:dbl)
        n42 = xnode "Invoke Method"("FPGA VI Reference In"=w281, "error in"=w272, "IRQ Number(s)"=w267) -> ("FPGA VI Reference Out"=w280:refnum<k20>, "error out"=w279:errorcluster)
        n43 = Number To Decimal String(number=w274) -> (decimal integer string=w273:string)  [unwired: 1 in]
        n44 = xnode "Invoke Method"("FPGA VI Reference In"=w280, "error in"=w279, "Number of Elements"=w277, "Timeout (ms)"="FIFO Timeout setting (ms)  2") -> ("FPGA VI Reference Out"=w278:refnum<k20>, "Data"=w269:u16[], "Elements Remaining"=→"Elements Remaining 6":u32)  [unwired: 1 out]
        "Raw Data 2" <- w269
        n45 = TDMS Write(0:w271, 7:w273, 9:w269) -> (4:w270:refnum<k34>)  [unwired: 3 in, 3 out]
      }
    }
    n46 = case shown="True" w182 {
      tunnel: w187 -> [w286 w290]
      tunnel: w186 -> [_ w291]
      tunnel: [w286 w300] -> w185
      tunnel: w91 -> [_ _]
      tunnel: w181 -> [w287 w298]
      tunnel: [w287 w297] -> w180
      tunnel: w166 -> [w285 w295]
      tunnel: [w285 w294] -> w165
      tunnel: [w282 w293] -> w133
      tunnel: w93 -> [_ w289]
      tunnel: w91 -> [_ w288]
      frame False {
        n47 = Initialize Array(0.0 ("element"), 768 ("dimension size")) -> (w282:dbl[])
      }
      frame True {
        n48 = Increment(x=w298) -> (x+1=w297:dbl)
        n49 = xnode "Invoke Method"("FPGA VI Reference In"=w290, "IRQ Number(s)"=w289) -> ()  [unwired: 1 in, 2 out]
        n50 = Number To Decimal String(number=w297) -> (decimal integer string=w296:string)  [unwired: 1 in]
        n51 = xnode "Invoke Method"("FPGA VI Reference In"=w290, "error in"=w291, "Number of Elements"=w288, "Timeout (ms)"="FIFO Timeout setting (ms)") -> ("FPGA VI Reference Out"=w300:refnum<k20>, "Data"=w293:u16[], "Elements Remaining"=→"Elements Remaining 5":u32)  [unwired: 1 out]
        "Raw Data" <- w293
        n52 = TDMS Write(0:w295, 7:w296, 9:w293) -> (4:w294:refnum<k34>)  [unwired: 3 in, 3 out]
      }
    }
    n53 = case shown="True" w171 {
      tunnel: w174 -> [w245 w260]
      tunnel: [w245 w257] -> _
      tunnel: w169 -> [_ w255]
      tunnel: w170 -> [w244 w253]
      tunnel: [w244 w252] -> w168
      tunnel: w173 -> [_ w250]
      tunnel: w162 -> [w243 w249]
      tunnel: [w243 w248] -> w161
      tunnel: [w240 w247] -> w131
      frame False {
        n54 = Initialize Array(0.0 ("element"), 768 ("dimension size")) -> (w240:dbl[])
      }
      frame True {
        n55 = Increment(x=w253) -> (x+1=w252:dbl)
        n56 = xnode "Invoke Method"("FPGA VI Reference In"=w260, "error in"=w250, "IRQ Number(s)"=2) -> ("FPGA VI Reference Out"=w259:refnum<k20>, "error out"=w258:errorcluster)
        n57 = Number To Decimal String(number=w252) -> (decimal integer string=w251:string)  [unwired: 1 in]
        n58 = xnode "Invoke Method"("FPGA VI Reference In"=w259, "error in"=w258, "Number of Elements"=w255, "Timeout (ms)"="FIFO Timeout setting (ms)  3") -> ("FPGA VI Reference Out"=w257:refnum<k20>, "Data"=w247:u16[], "Elements Remaining"=→"Elements Remaining 7":u32)  [unwired: 1 out]
        "Raw Data 3" <- w247
        n59 = TDMS Write(0:w249, 7:w251, 9:w247) -> (4:w248:refnum<k34>)  [unwired: 3 in, 3 out]
      }
    }
    n60 = case shown="True" w146 {
      tunnel: w154 -> [w224 w239]
      tunnel: [w224 w236] -> _
      tunnel: w151 -> [_ w234]
      tunnel: w149 -> [w223 w232]
      tunnel: [w223 w231] -> w148
      tunnel: w153 -> [_ w229]
      tunnel: w150 -> [w222 w228]
      tunnel: [w222 w227] -> w147
      tunnel: [w219 w226] -> w130
      frame False {
        n61 = Initialize Array(0.0 ("element"), 768 ("dimension size")) -> (w219:dbl[])
      }
      frame True {
        n62 = Increment(x=w232) -> (x+1=w231:dbl)
        n63 = xnode "Invoke Method"("FPGA VI Reference In"=w239, "error in"=w229, "IRQ Number(s)"=3) -> ("FPGA VI Reference Out"=w238:refnum<k20>, "error out"=w237:errorcluster)
        n64 = Number To Decimal String(number=w231) -> (decimal integer string=w230:string)  [unwired: 1 in]
        n65 = xnode "Invoke Method"("FPGA VI Reference In"=w238, "error in"=w237, "Number of Elements"=w234, "Timeout (ms)"="FIFO Timeout setting (ms)  4") -> ("FPGA VI Reference Out"=w236:refnum<k20>, "Data"=w226:u16[], "Elements Remaining"=→"Elements Remaining 8":u32)  [unwired: 1 out]
        "Raw Data 4" <- w226
        n66 = TDMS Write(0:w228, 7:w230, 9:w226) -> (4:w227:refnum<k34>)  [unwired: 3 in, 3 out]
      }
    }
    n67 = Compound Arithmetic op=ADD(w145, w137, w138, w139, w140, w141, w142, w143, w144, w111) -> (w109:dbl[])
    n68 = case shown="3" "control" {
      tunnel: [w215 w216 w217 w218] -> w128
      tunnel: w133 -> [w215 _ _ _]
      tunnel: w132 -> [_ w216 _ _]
      tunnel: w131 -> [_ _ w217 _]
      tunnel: w130 -> [_ _ _ w218]
      frame 1, Default {
      }
      frame 2 {
      }
      frame 3 {
      }
      frame 4 {
      }
    }
    n69 = Initialize Array(10.0 ("element"), 768 ("dimension size")) -> (w134:dbl[])
    n70 = Divide(x=w109, y=w134) -> (x/y=w110:dbl[])
    n71 = Subtract(x=w128, y=w110) -> (x-y=w126:dbl[])
    "Subtraction-10 frames average" <- w126
    n72 = Multiply(x=w126, y=-1.0) -> (x*y=w112:dbl[])
    n73 = for {
      N: 768 -> [_]
      tunnel: w112 -> [w214] mode=indexing
      tunnel: [w210] -> w113 mode=indexing
      w211 = 0.0 ("y")
      n74 = Subtract(x=w214, y="threshold 3") -> (x-y=w212:dbl)
      n75 = Greater?(x=w212, y=w211) -> (0:w213:bool)
      n76 = Select(t=w212, s=w213, f=w211) -> (s? t:f=w210:dbl)
    }
    n77 = call-poly <vilib>:"Butterworth Filter.vi"("order"="order", "low cutoff freq: fl"="low cutoff freq: fl", "high cutoff freq: fh"="high cutoff freq: fh", "sampling freq: fs"="sampling freq: fs", "X"=w113) -> ("Filtered X"=w119:dbl[])  [unwired: 3 in, 1 out]
    n78 = for {
      N: 768 -> [_]
      tunnel: w119 -> [w206] mode=indexing
      tunnel: [w207] -> w118 mode=indexing
      tunnel: [w206] -> w117 mode=indexing
      i -> [w208]
      n79 = Multiply(x=w206, y=w208) -> (x*y=w207:dbl)
    }
    n80 = Add Array Elements(numeric array=w118) -> (sum=w116:dbl)
    n81 = Add Array Elements(numeric array=w117) -> (sum=w115:dbl)
    n82 = Divide(x=w116, y=w115) -> (x/y=→"Fly real-time location/center mass":dbl)
    n83 = node-c288() -> ()  [unwired: 1 in, 1 out]
  }
  n84 = while {
    tunnel: w5 -> [w336]
    tunnel: [w335] -> _
    tunnel: w5 -> [w331]
    tunnel: [w330] -> _
    tunnel: w5 -> [w316]
    tunnel: w5 -> [w315]
    tunnel: [w314] -> _
    tunnel: [w313] -> _
    stop <- "LED stop" stop-if-true
    n85 = Subtract(x=4000.0, y="LED High Period (ticks) J5") -> (x-y=w327:dbl)
    n86 = Subtract(x=4000.0, y="LED High Period (ticks) J4") -> (x-y=w323:dbl)
    n87 = Subtract(x=4000.0, y="LED High Period (ticks) J1") -> (x-y=w333:dbl)
    n88 = Subtract(x=4000.0, y="LED High Period (ticks) J8") -> (x-y=w319:dbl)
    n89 = xnode "Read/Write Control"("FPGA VI Reference In"=w316, "High Period (ticks) J4"="LED High Period (ticks) J4", "Low Period (ticks) J4"=w323, "Apply J4"=TRUE, "Output Enable J4"=TRUE) -> ("FPGA VI Reference Out"=w314:refnum<k20>, "Timed Out? J4"=→"FIFO Timed Out? J4":bool)  [unwired: 1 in, 1 out]
    n90 = xnode "Read/Write Control"("FPGA VI Reference In"=w331, "Half-clock time J5"="LED High Period (ticks) J5", "Low Period (ticks) J5"=w327, "Apply J5"=TRUE, "Output Enable J5"=TRUE) -> ("FPGA VI Reference Out"=w330:refnum<k20>, "Timed Out? J5"=→"FIFO Timed Out? J5":bool)  [unwired: 1 in, 1 out]
    n91 = xnode "Read/Write Control"("FPGA VI Reference In"=w336, "High Period (ticks) J1"="LED High Period (ticks) J1", "Low Period (ticks) J1"=w333, "Apply J1"=TRUE, "Output Enable J1"=TRUE) -> ("FPGA VI Reference Out"=w335:refnum<k20>, "Timed Out? J1"=→"FIFO Timed Out? J1":bool)  [unwired: 1 in, 1 out]
    n92 = xnode "Read/Write Control"("FPGA VI Reference In"=w315, "High Period (ticks) J8"="LED High Period (ticks) J8", "Low Period (ticks) J8"=w319, "Apply J8"=TRUE, "Output Enable J8"=TRUE) -> ("FPGA VI Reference Out"=w313:refnum<k20>, "Timed Out? J8"=→"FIFO Timed Out? J8":bool)  [unwired: 1 in, 1 out]
  }
  n93 = TDMS Close(11:w59) -> ()  [unwired: 1 in, 2 out]
  n94 = TDMS Close(11:w11) -> ()  [unwired: 1 in, 2 out]
  n95 = TDMS Close(11:w31) -> ()  [unwired: 1 in, 2 out]
  n96 = TDMS Close(11:w33) -> ()  [unwired: 1 in, 2 out]
  n97 = node-c288(w89) -> ()  [unwired: 1 out]
  "Path 2" <- "Path"
